vi "Autonomous Independent.vi"   [LabVIEW 2020]
doc: "This VI is called when autonomous begins, and will automatically be terminated when autonomous ends. You can carry out timed or sensor driven robot movement independently without needing to return to the caller."
uses:
  <vilib>/Rock Robotics/WPI/SafetyOutput/WPI_SafetyOutputConfigMenu.ctl
  <vilib>/Rock Robotics/WPI/Solenoid/WPI_SolenoidValue.ctl
  <vilib>/Rock Robotics/WPI/ThirdParty/REV Robotics/REVLib/Typedef/Spark MAX Control Type.ctl
  <vilib>/Rock Robotics/WPI/Utilities/WPI_GetSetVariantRefNum.vi
  <vilib>/Rock Robotics/Network Tables/NT Read String.vi
  <vilib>/Rock Robotics/Network Tables/NT Write Numeric Array.vi
  <vilib>/Rock Robotics/Network Tables/NT Read Number.vi
  Auto Variables.vi
  <vilib>/Rock Robotics/WPI/Solenoid/WPI_SolenoidSetEnum.vi
  Global Shooter Speed.vi
panel:
  # "Be sure to right-click and choose Data Operations>>Make Current Value default if you want to save the array values with the VI"
types:
  T1 = typedef "WPI_SafetyOutputConfigMenu.ctl" = enum16{"Enable", "Disable"}
  T2 = typedef "WPI_JoystickDevRef.ctl" = cluster{"Device":T3}
  T3 = typedef "WPI_JoystickDeviceEnum.ctl" = enum16{"USB 0", "USB 1", "USB 2", "USB 3", "USB 4", "USB 5"}
  T4 = typedef "WPI_RobotDriveDevRef.ctl" = cluster{"DevStatus":errorcluster, "Motors[]":T5[], "Square Inputs":bool, "Max Output":dbl}
  T5 = typedef "WPI_MotorControlDeviceRef.ctl" = cluster{"DeviceStatus":errorcluster, "Type":T6, "PWM":cluster{"PWM Channel":T7, "DeadBand":T8}, "CAN":cluster{"Device Number":u8, "SetOutput VI Ref":variant, "GetOutput VI Ref":variant, "Enable VI Ref":variant, "Disable VI Ref":variant, "Data":variant}, "Invert":bool, "DIO PWM":cluster{"PWM \"Enable\" Channel":T7, "DIOChannel":T9, "PWM Rate":dbl}}
  T6 = typedef "WPI_MotorControlType.ctl" = enum16{"PWM", "CAN", "DIO PWM"}
  T7 = typedef "FPGA_DIOPWMChannel.ctl" = enum8{"PWM 0", "PWM 1", "PWM 2", "PWM 3", "PWM 4", "PWM 5", "PWM 6", "PWM 7", "PWM 8", "PWM 9", "PWM MXP 0", "PWM MXP 1", "PWM MXP 2", "PWM MXP 3", "PWM MXP 4", "PWM MXP 5", "PWM MXP 6", "PWM MXP 7", "PWM MXP 8", "PWM MXP 9", "Invalid"}
  T8 = typedef "WPI_PWMDeadband.ctl" = cluster{"Name":string, "maxPositivePwm":i32, "minPositivePwm":i32, "centerPwm":i32, "maxNegativePwm":i32, "minNegativePwm":i32, "angularRange":u16}
  T9 = typedef "FPGA_DIOChannel.ctl" = enum8{"DIO 0", "DIO 1", "DIO 2", "DIO 3", "DIO 4", "DIO 5", "DIO 6", "DIO 7", "DIO 8", "DIO 9", "DIO MXP 0", "DIO MXP 1", "DIO MXP 2", "DIO MXP 3", "DIO MXP 4", "DIO MXP 5", "DIO MXP 6", "DIO MXP 7", "DIO MXP 8", "DIO MXP 9", "DIO MXP 10", "DIO MXP 11", "DIO MXP 12", "DIO MXP 13", "DIO MXP 14", "DIO MXP 15", "SPI Port CS1", "SPI Port CS2", "SPI Port CS3", "SPI Port MISO", "SPI Port MOSI", "Invalid"}
  T10 = typedef "WPI_SolenoidValue.ctl" = enum16{"Off", "On", "Forward", "Reverse"}
  T11 = typedef "Spark MAX Control Type.ctl" = enum16{"Percent VBus", "Voltage", "Velocity", "Position", "Smart Motion", "Current", "Smart Velocity"}
  T12 = typedef "WPI_SolenoidDevRef.ctl" = cluster{"DevStatus":errorcluster, "Pneumatics Control Module":u8, "Forward Solenoid Channel":T13, "Reverse Solenoid Channel":T13}
  T13 = typedef "WPI_SolenoidChannel.ctl" = enum8{"Solenoid 0", "Solenoid 1", "Solenoid 2", "Solenoid 3", "Solenoid 4", "Solenoid 5", "Solenoid 6", "Solenoid 7", "Solenoid 8", "Solenoid 9", "Solenoid 10", "Solenoid 11", "Solenoid 12", "Solenoid 13", "Solenoid 14", "Solenoid 15", "Invalid"}
  T14 = typedef "WPI_GyroDevRef.ctl" = cluster{"DevStatus":errorcluster, "Analog Channel":T15, "Gain (VoltsPerDegree/Second)":dbl, "Gyro Type":enum16{"Analog", "XRS450"}, "Handle":i32, "SPI Bus":T16, "Device Found":bool, "Sample Rate":dbl, "Calibrate On Open":bool, "Offset":dbl}
  T15 = typedef "FPGA_AIChannel.ctl" = enum8{"AI 0", "AI 1", "AI 2", "AI 3", "AI MXP 0", "AI MXP 1", "AI MXP 2", "AI MXP 3", "Invalid"}
  T16 = typedef "spi_bus.ctl" = enum16{"SPI On-Board, CS0", "SPI On-Board, CS1", "SPI On-Board, CS2", "SPI On-Board, CS3", "SPI MXP", "Invalid"}
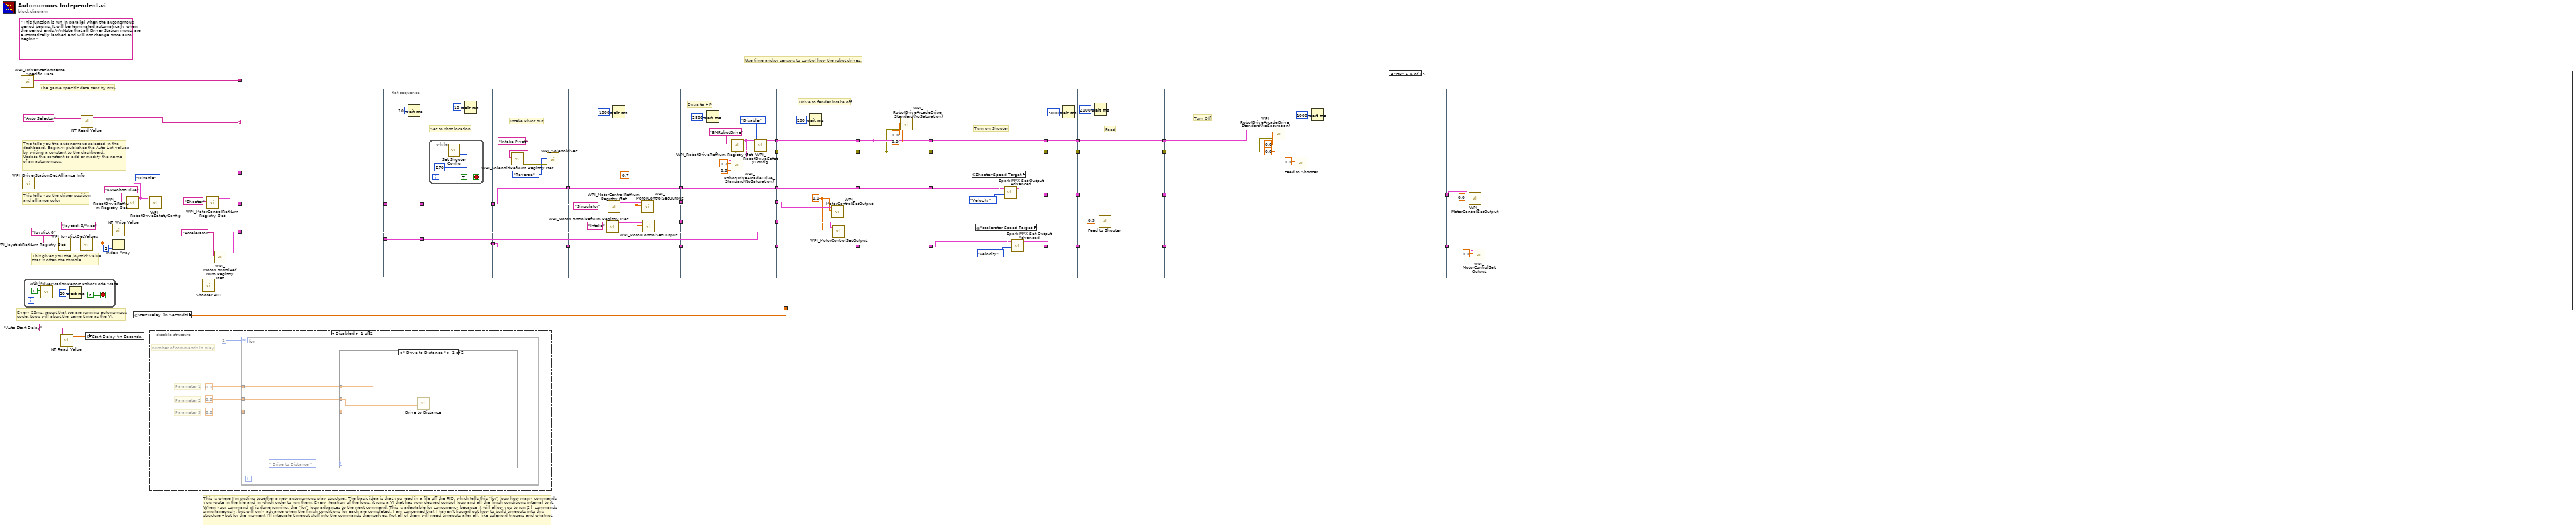
[diagram p0: block diagram]
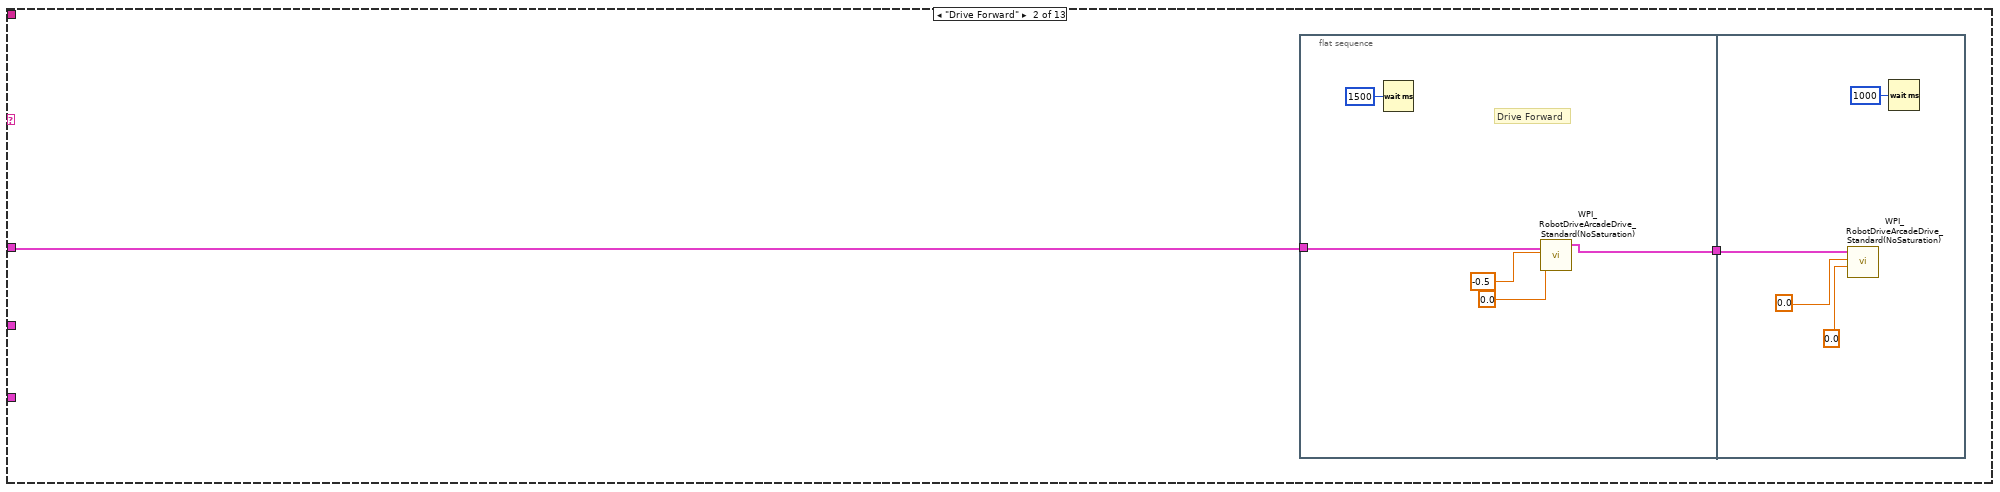
[diagram p5: hidden frame]
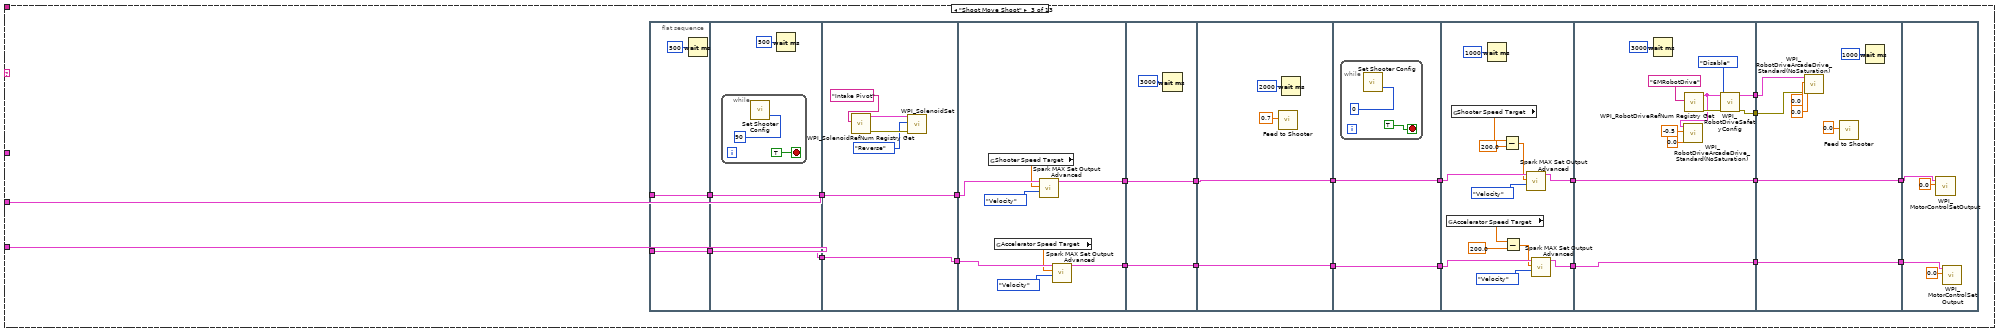
[diagram p6: hidden frame]
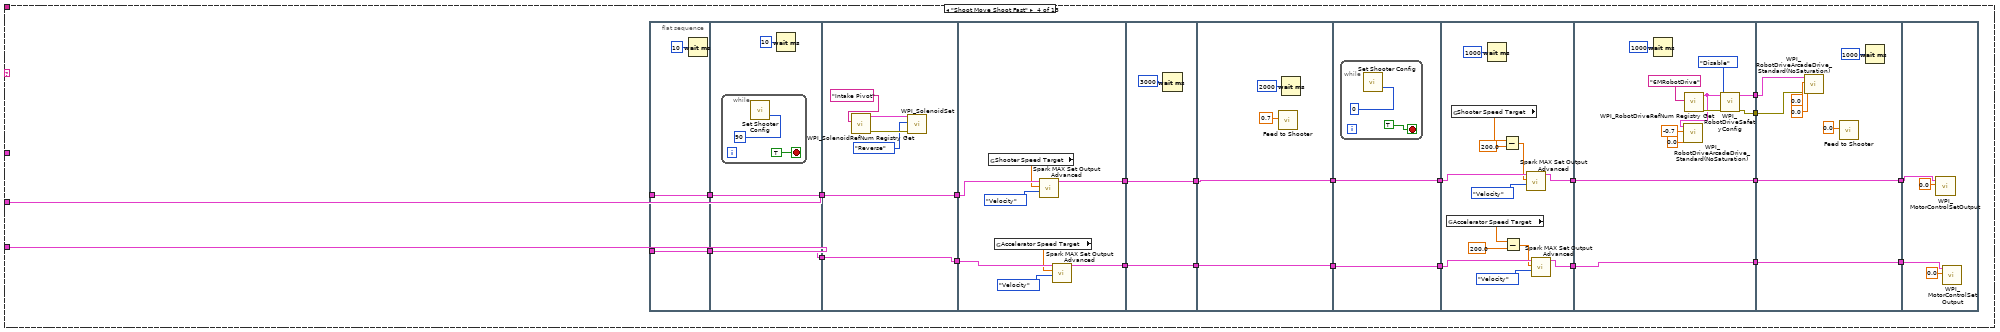
[diagram p7: hidden frame]
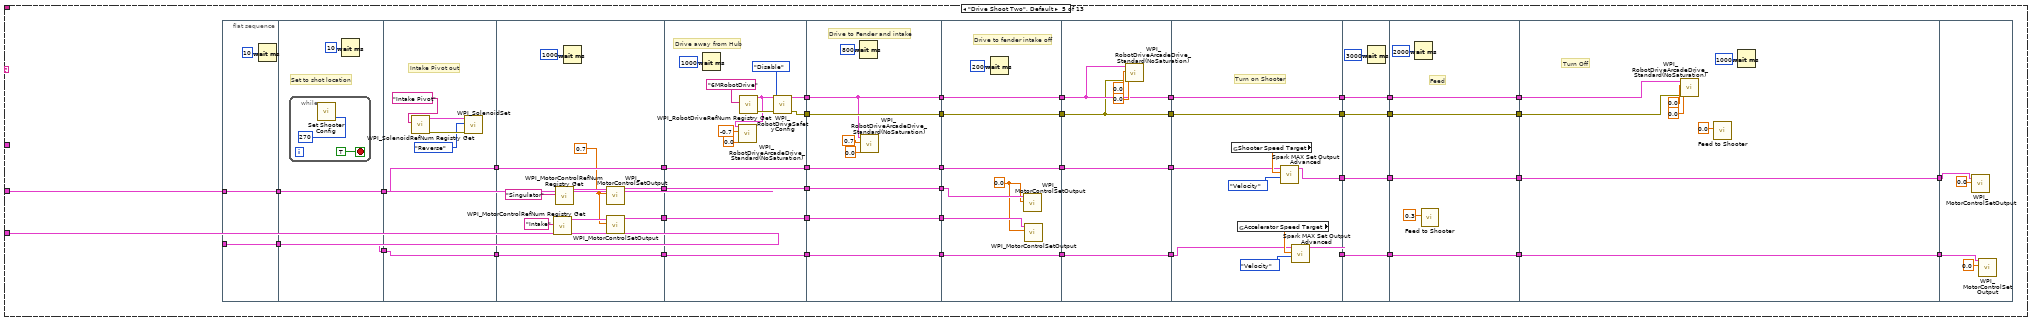
[diagram p8: hidden frame]
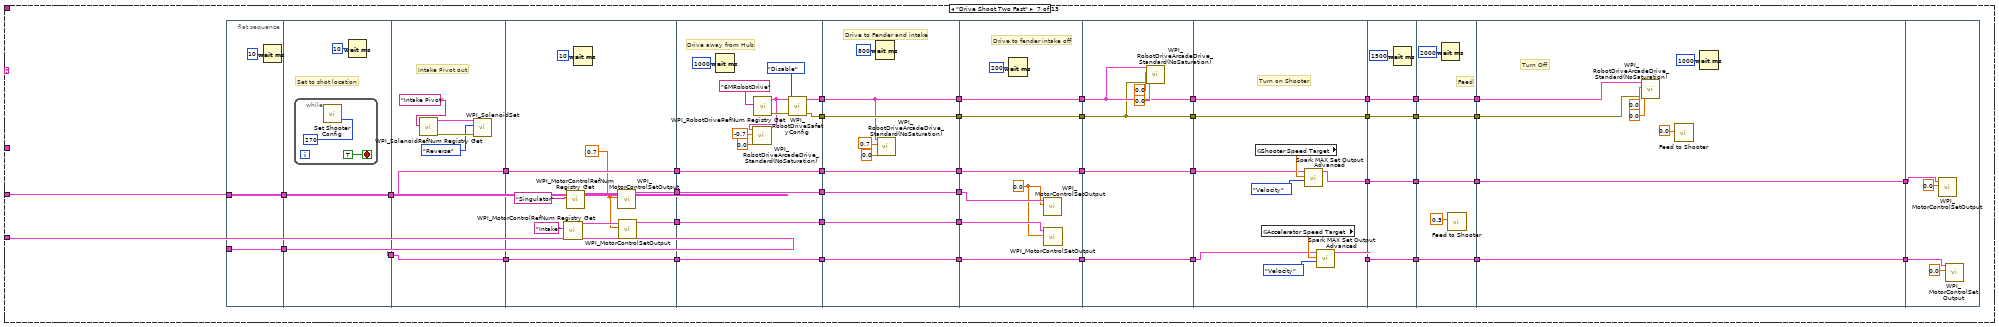
[diagram p9: hidden frame]
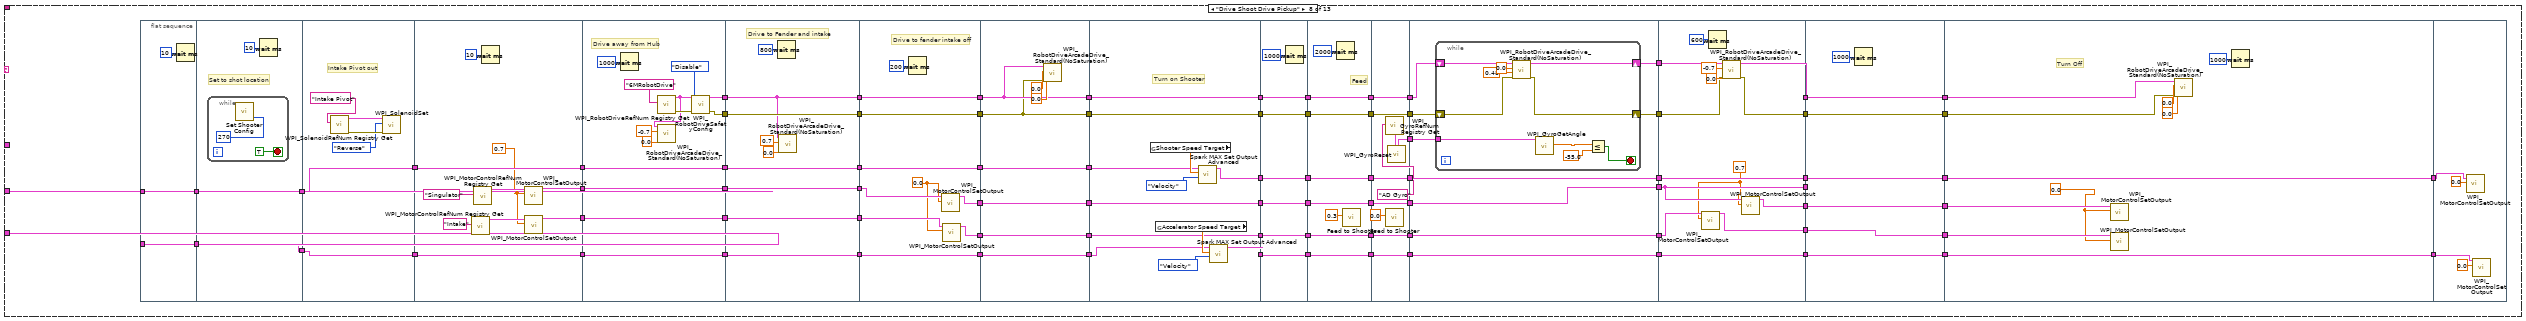
[diagram p10: hidden frame]
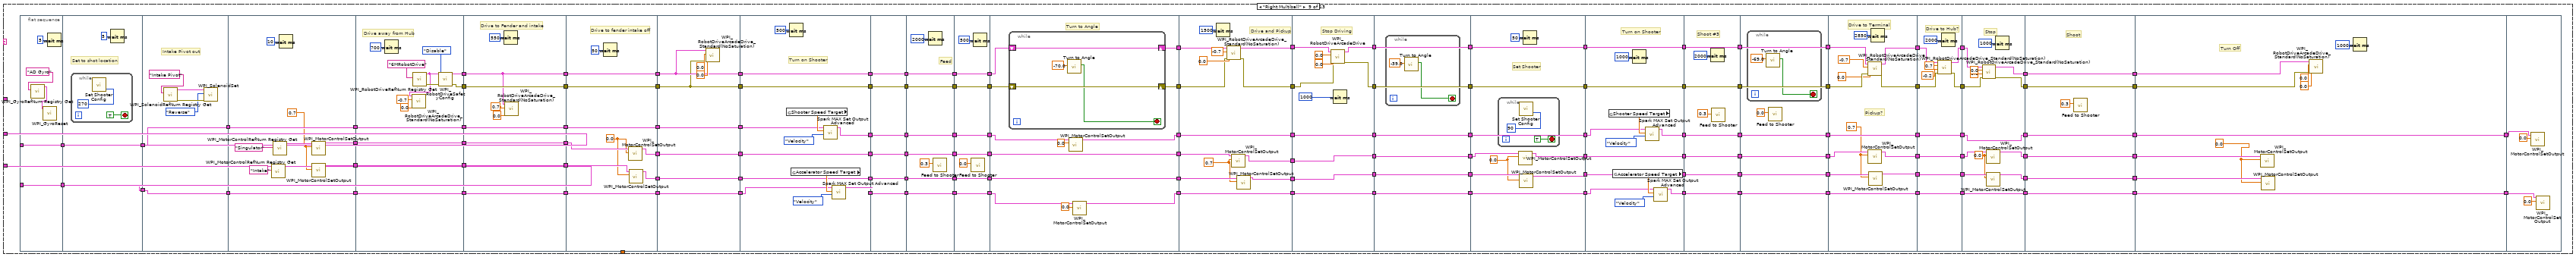
[diagram p11: hidden frame]
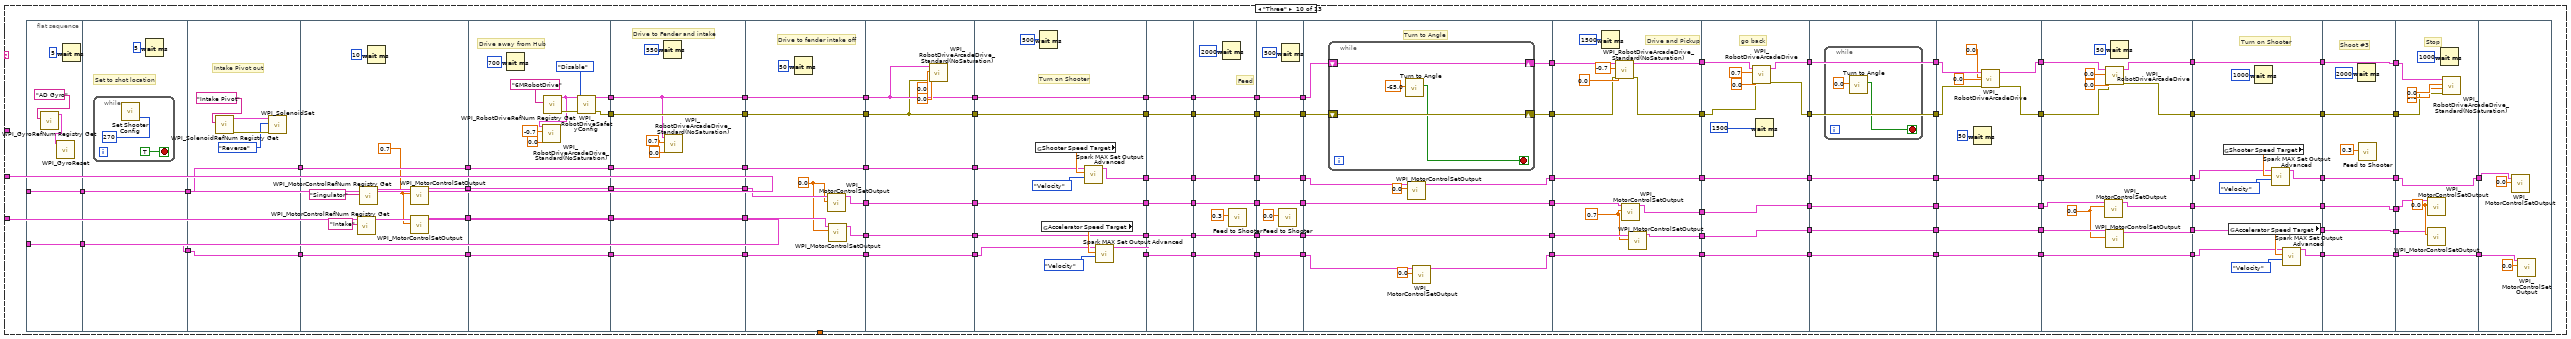
[diagram p12: hidden frame]
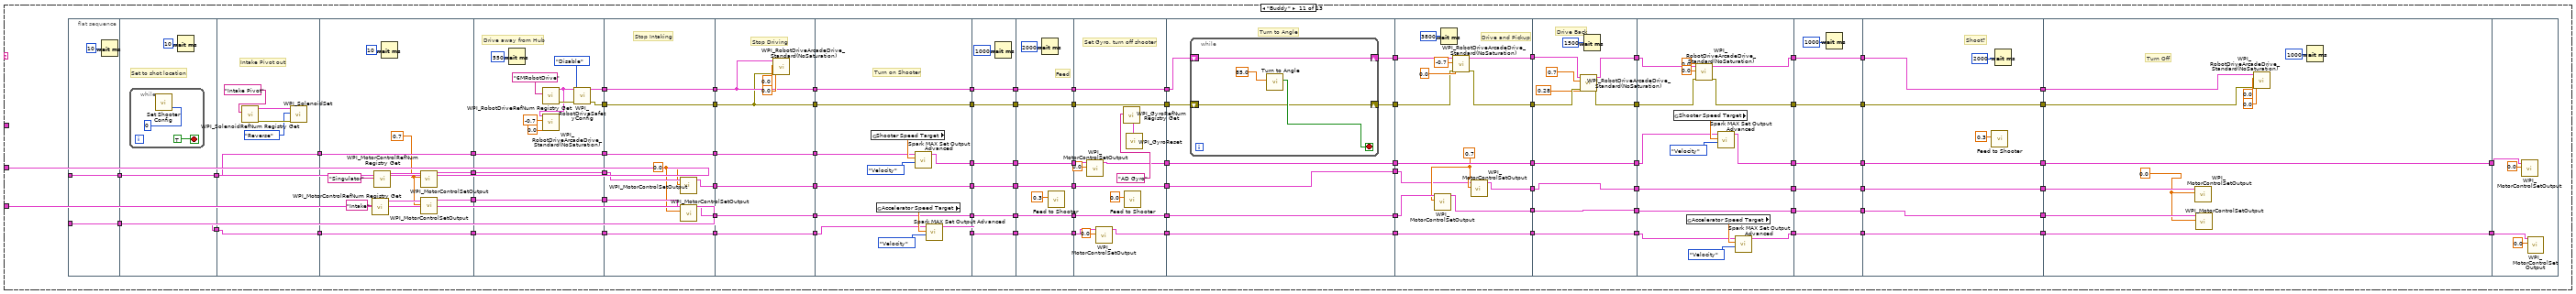
[diagram p13: hidden frame]
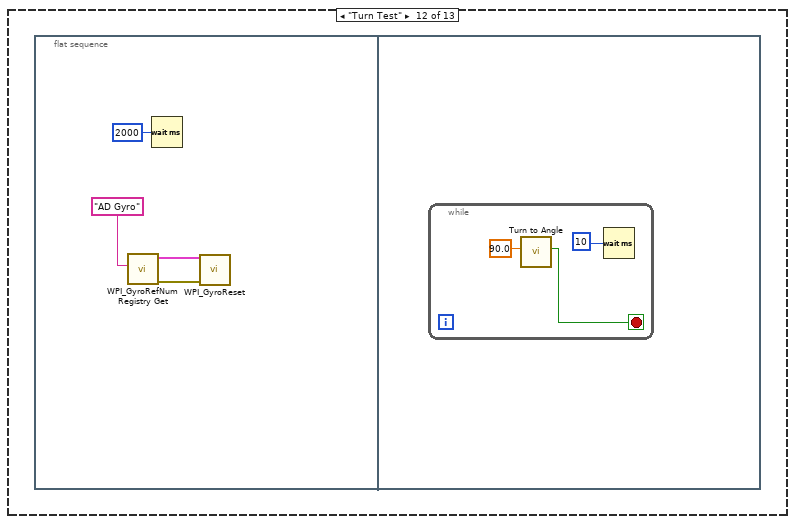
[diagram p14: hidden frame]
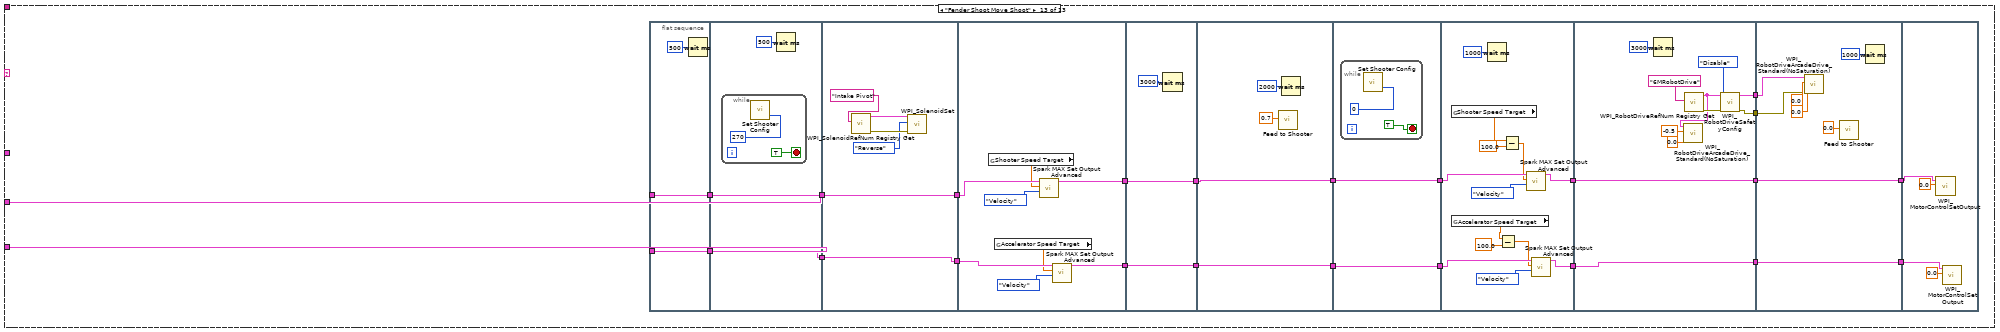
[diagram p15: hidden frame]
diagram:
  (unwired) "This function is run in parallel when the autonomous period begins. It will be terminated automatically when the period ends.\n\nNote that all Driver Station inputs are automatically latched and will not change once auto begins."
  # "This is where I'm putting together a new autonomous play structure. The basic idea is that you read in a file off the RIO, which tells this \"for\" loop how many commands\nyou wrote in the file and in which order to run them. Every iteration of the loop, it runs a VI that has your desired control loop and all the finish conditions internal to it.\nWhen your command VI is done running, the \"for\" loop advances to the next command. This is adaptable for concurrency because it will allow you to run 2+ commands\nsimultaneously, but will only advance when the finish conditions for each are completed. I am concerned that I haven't figured out how to build timeouts into this\nstructure - but for the moment I'll integrate timeout stuff into the commands themselves. Not all of them will need timeouts after all, like solenoid triggers and whatnot."
  # "The game specific data sent by FMS"
  # "This tells you the autonomous selected in the \ndashboard. Begin.vi publishes the Auto List values\nby writing a constant to the dashboard.\nUpdate the constant to add or modify the name\nof an autonomous."
  # "Every 20ms, report that we are running autonomous\ncode. Loop will abort the same time as the VI."
  # "This gives you the joystick value\nthat is often the throttle"
  # "Use time and/or sensors to control how the robot drives."
  # "This tells you the driver position\nand alliance color"
  n1 = call <vilib>:"WPI_DriverStationGame Specific Data.vi"() -> ("Game Specific Data"=w13:string)  [unwired: 11 in]
  n2 = call <vilib>:"WPI_DriverStationGet Alliance Info.vi"() -> ()  [unwired: 12 out]
  n3 = while {
    stop <- FALSE stop-if-true
    n4 = call <vilib>:"WPI_DriverStationReport Robot Code State.vi"("Autonomous"=TRUE) -> ()  [unwired: 10 in, 1 out]
    n5 = Wait (ms)(milliseconds to wait=u32 20) -> ()  [unwired: 1 out]
  }
  n6 = call <vilib>:"WPI_JoystickRefNum Registry Get.vi"("refnum name"="Joystick 0") -> ("JoystickDevRef"=w18:T2)  [unwired: 1 in, 9 out]
  n7 = call-poly <vilib>:"NT Read Value.vi"("Name"="Auto Start Delay") -> ("Numeric"=w10:dbl)  [unwired: 9 in, 1 out]
  n8 = call <vilib>:"WPI_JoystickGetValues.vi"("JoystickDevRef"=w18) -> ("Axes"=w15:dbl[])  [unwired: 6 in, 4 out]
  n9 = call-poly <vilib>:"NT Read Value.vi"("Name"="Auto Selector") -> ("String"=w1:string)  [unwired: 9 in, 1 out]
  n10 = global write "Auto Variables.vi" "Start Delay (in Seconds)"(w10) -> ()
  n11 = call-poly <vilib>:"NT Write Value.vi"("Numeric Array"=w15, "Name"="Joystick 0/Axes") -> ()  [unwired: 9 in, 1 out]
  n12 = Index Array(array=w15, index=2) -> ()  [unwired: 1 out]
  n13 = call <vilib>:"WPI_RobotDriveRefNum Registry Get.vi"("refnum name"="6MRobotDrive") -> ("error out"=w9:errorcluster, "RobotDriveDevRef"=w6:T4)  [unwired: 1 in, 8 out]
  n14 = global read "Auto Variables.vi" "Start Delay (in Seconds)"() -> (w12:dbl)
  n15 = disable-structure shown="Disabled" {
    frame Disabled {
      # "Parameter 3"
      # "Parameter 2"
      # "Parameter 1"
      # "number of commands in play"
      n16 = for {
        N: 1 -> [_]
        tunnel: 0.0 -> [w30]
        tunnel: 0.0 -> [w29]
        tunnel: 0.0 -> [w28]
        n17 = case shown="\" Drive to Distance \"" enum16{"No-op", " Drive to Distance "}." Drive to Distance " {
          tunnel: w30 -> [_ w32]
          tunnel: w29 -> [_ w31]
          tunnel: w28 -> [_ _]
          frame "No-op", Default {
          }
          frame " Drive to Distance " {
            n18 = call "Drive to Distance.vi"("Acceptable Error (in)"=w31, "Target in Inches"=w32) -> ()  [unwired: 9 in, 1 out]
          }
        }
      }
    }
    frame Enabled {
    }
  }
  n19 = call <vilib>:"WPI_RobotDriveSafetyConfig.vi"("error in (no error)"=w9, "mode"=WPI_SafetyOutputConfigMenu."Disable", "RobotDriveDevRef"=w6) -> ()  [unwired: 7 in, 2 out]
  n20 = call "Shooter PID.vi"() -> ()  [unwired: 12 in]
  n21 = call <vilib>:"WPI_MotorControlRefNum Registry Get.vi"("refnum name"="Shooter") -> ("MotorControlDevRef"=w5:T5)  [unwired: 9 in, 1 out]
  n22 = call <vilib>:"WPI_MotorControlRefNum Registry Get.vi"("refnum name"="Accelerator") -> ("MotorControlDevRef"=w4:T5)  [unwired: 9 in, 1 out]
  n23 = case shown="\"HP\"" w1 {
    tunnel: w13 -> [_ _ _ _ _ _ _ _ _ _ _ _ _]
    tunnel: w12 -> [_ _ _ _ _ _ _ _ _ _ _ _ _]
    tunnel: w6 -> [_ w34 _ _ _ _ _ _ _ _ _ _ _]
    tunnel: w5 -> [_ _ w64 w157 w274 w407 w537 w712 w1001 w1363 w1665 _ w1870]
    tunnel: w4 -> [_ _ w60 w153 w272 w405 w535 w710 w999 w1361 w1663 _ w1866]
    frame "Do Nothing" {
    }
    frame "Drive Forward" {
      n24 = flat-sequence {
        tunnel: w34 -> [w36]
        tunnel: [w35] -> w33
        tunnel: w33 -> [w40]
        frame #0 {
          # "Drive Forward"
          n25 = Wait (ms)(milliseconds to wait=u32 1500) -> ()  [unwired: 1 out]
          n26 = call <vilib>:"WPI_RobotDriveArcadeDrive_Standard(NoSaturation).vi"("Y axis value"=0.0, "X axis value"=-0.5, "RobotDriveDevRef"=w36) -> ("RobotDriveDevRef"=w35:T4)  [unwired: 1 in, 7 out]
        }
        frame #1 {
          n27 = call <vilib>:"WPI_RobotDriveArcadeDrive_Standard(NoSaturation).vi"("Y axis value"=0.0, "X axis value"=0.0, "RobotDriveDevRef"=w40) -> ()  [unwired: 1 in, 8 out]
          n28 = Wait (ms)(milliseconds to wait=u32 1000) -> ()  [unwired: 1 out]
        }
      }
    }
    frame "Shoot Move Shoot" {
      n29 = flat-sequence {
        tunnel: w60 -> [w69]
        tunnel: w64 -> [w70]
        tunnel: [w70] -> w45
        tunnel: [w69] -> w44
        tunnel: [w72] -> w65
        tunnel: [w71] -> w61
        tunnel: w45 -> [w72]
        tunnel: w44 -> [w71]
        tunnel: w65 -> [w77]
        tunnel: [w77] -> w63
        tunnel: [w76] -> w62
        tunnel: w61 -> [w76]
        tunnel: w63 -> [w89]
        tunnel: w62 -> [w88]
        tunnel: [w83] -> w49
        tunnel: [w82] -> w47
        tunnel: w49 -> [w92]
        tunnel: [w92] -> w48
        tunnel: w47 -> [w91]
        tunnel: [w91] -> w46
        tunnel: [w95] -> w53
        tunnel: w48 -> [w95]
        tunnel: [w94] -> w51
        tunnel: w46 -> [w94]
        tunnel: w53 -> [w98]
        tunnel: [w98] -> w52
        tunnel: w51 -> [w97]
        tunnel: [w97] -> w50
        tunnel: w52 -> [w111]
        tunnel: [w110] -> w57
        tunnel: w50 -> [w108]
        tunnel: [w107] -> w56
        tunnel: [w118] -> w67
        tunnel: [w117] -> w66
        tunnel: w57 -> [w115]
        tunnel: w56 -> [w114]
        tunnel: [w115] -> w59
        tunnel: [w114] -> w58
        tunnel: w67 -> [w129]
        tunnel: w66 -> [w128]
        tunnel: w59 -> [w125]
        tunnel: w58 -> [w126]
        tunnel: [w126] -> w55
        tunnel: [w125] -> w54
        tunnel: w55 -> [w135]
        tunnel: w54 -> [w133]
        frame #0 {
          n30 = Wait (ms)(milliseconds to wait=u32 500) -> ()  [unwired: 1 out]
        }
        frame #1 {
          n31 = while {
            stop <- TRUE stop-if-true
            n32 = call "Set Shooter Config.vi"("POV Joystick Input"=90) -> ()  [unwired: 3 in]
          }
          n33 = Wait (ms)(milliseconds to wait=u32 500) -> ()  [unwired: 1 out]
        }
        frame #2 {
          n34 = call <vilib>:"WPI_SolenoidRefNum Registry Get.vi"("refnum name"="Intake Pivot") -> ("error out"=w81:errorcluster, "SolenoidDevRef"=w80:T12)  [unwired: 9 in]
          n35 = call-poly <vilib>:"WPI_SolenoidSet.vi"("error in (no error)"=w81, "Value"=WPI_SolenoidValue."Reverse", "SolenoidDevRef"=w80) -> ()  [unwired: 7 in, 2 out]
        }
        frame #3 {
          n36 = global read "Global Shooter Speed.vi" "Shooter Speed Target"() -> (w86:dbl)
          n37 = global read "Global Shooter Speed.vi" "Accelerator Speed Target"() -> (w84:dbl)
          n38 = call <vilib>:"Spark MAX Set Output Advanced.vi"("Control Mode"=Spark_MAX_Control_Type."Velocity", "Setpoint"=w86, "MotorControlDevRef"=w89) -> ("MotorControlDevRef"=w83:T5)  [unwired: 7 in, 1 out]
          n39 = call <vilib>:"Spark MAX Set Output Advanced.vi"("Control Mode"=Spark_MAX_Control_Type."Velocity", "Setpoint"=w84, "MotorControlDevRef"=w88) -> ("MotorControlDevRef"=w82:T5)  [unwired: 7 in, 1 out]
        }
        frame #4 {
          n40 = Wait (ms)(milliseconds to wait=u32 3000) -> ()  [unwired: 1 out]
        }
        frame #5 {
          n41 = call "Feed to Shooter.vi"("Feed Input"=0.7) -> ()  [unwired: 11 in]
          n42 = Wait (ms)(milliseconds to wait=u32 2000) -> ()  [unwired: 1 out]
        }
        frame #6 {
          n43 = while {
            stop <- TRUE stop-if-true
            n44 = call "Set Shooter Config.vi"("POV Joystick Input"=0) -> ()  [unwired: 3 in]
          }
        }
        frame #7 {
          n45 = global read "Global Shooter Speed.vi" "Accelerator Speed Target"() -> (w102:dbl)
          n46 = global read "Global Shooter Speed.vi" "Shooter Speed Target"() -> (w106:dbl)
          n47 = Wait (ms)(milliseconds to wait=u32 1000) -> ()  [unwired: 1 out]
          n48 = Subtract(x=w106, y=200.0) -> (x-y=w104:dbl)
          n49 = Subtract(x=w102, y=200.0) -> (x-y=w103:dbl)
          n50 = call <vilib>:"Spark MAX Set Output Advanced.vi"("Control Mode"=Spark_MAX_Control_Type."Velocity", "Setpoint"=w104, "MotorControlDevRef"=w111) -> ("MotorControlDevRef"=w110:T5)  [unwired: 7 in, 1 out]
          n51 = call <vilib>:"Spark MAX Set Output Advanced.vi"("Control Mode"=Spark_MAX_Control_Type."Velocity", "Setpoint"=w103, "MotorControlDevRef"=w108) -> ("MotorControlDevRef"=w107:T5)  [unwired: 7 in, 1 out]
        }
        frame #8 {
          n52 = Wait (ms)(milliseconds to wait=u32 3000) -> ()  [unwired: 1 out]
          n53 = call <vilib>:"WPI_RobotDriveRefNum Registry Get.vi"("refnum name"="6MRobotDrive") -> ("error out"=w121:errorcluster, "RobotDriveDevRef"=w120:T4)  [unwired: 1 in, 8 out]
          n54 = call <vilib>:"WPI_RobotDriveArcadeDrive_Standard(NoSaturation).vi"("Y axis value"=0.0, "X axis value"=-0.5, "RobotDriveDevRef"=w120) -> ()  [unwired: 1 in, 8 out]
          n55 = call <vilib>:"WPI_RobotDriveSafetyConfig.vi"("error in (no error)"=w121, "mode"=WPI_SafetyOutputConfigMenu."Disable", "RobotDriveDevRef"=w120) -> ("error out"=w117:errorcluster, "RobotDriveDevRef"=w118:T4)  [unwired: 7 in]
        }
        frame #9 {
          n56 = call <vilib>:"WPI_RobotDriveArcadeDrive_Standard(NoSaturation).vi"("error in (no error)"=w128, "Y axis value"=0.0, "X axis value"=0.0, "RobotDriveDevRef"=w129) -> ()  [unwired: 8 out]
          n57 = call "Feed to Shooter.vi"("Feed Input"=0.0) -> ()  [unwired: 11 in]
          n58 = Wait (ms)(milliseconds to wait=u32 1000) -> ()  [unwired: 1 out]
        }
        frame #10 {
          n59 = call <vilib>:"WPI_MotorControlSetOutput.vi"("Output"=0.0, "MotorControlDevRef"=w133) -> ()  [unwired: 7 in, 3 out]
          n60 = call <vilib>:"WPI_MotorControlSetOutput.vi"("Output"=0.0, "MotorControlDevRef"=w135) -> ()  [unwired: 7 in, 3 out]
        }
      }
    }
    frame "Shoot Move Shoot Fast" {
      n61 = flat-sequence {
        tunnel: w153 -> [w162]
        tunnel: w157 -> [w163]
        tunnel: [w163] -> w138
        tunnel: [w162] -> w137
        tunnel: [w165] -> w158
        tunnel: [w164] -> w154
        tunnel: w138 -> [w165]
        tunnel: w137 -> [w164]
        tunnel: w158 -> [w170]
        tunnel: [w170] -> w156
        tunnel: [w169] -> w155
        tunnel: w154 -> [w169]
        tunnel: w156 -> [w182]
        tunnel: w155 -> [w181]
        tunnel: [w176] -> w142
        tunnel: [w175] -> w140
        tunnel: w142 -> [w185]
        tunnel: [w185] -> w141
        tunnel: w140 -> [w184]
        tunnel: [w184] -> w139
        tunnel: [w188] -> w146
        tunnel: w141 -> [w188]
        tunnel: [w187] -> w144
        tunnel: w139 -> [w187]
        tunnel: w146 -> [w191]
        tunnel: [w191] -> w145
        tunnel: w144 -> [w190]
        tunnel: [w190] -> w143
        tunnel: w145 -> [w204]
        tunnel: [w203] -> w150
        tunnel: w143 -> [w201]
        tunnel: [w200] -> w149
        tunnel: [w211] -> w160
        tunnel: [w210] -> w159
        tunnel: w150 -> [w208]
        tunnel: w149 -> [w207]
        tunnel: [w208] -> w152
        tunnel: [w207] -> w151
        tunnel: w160 -> [w222]
        tunnel: w159 -> [w221]
        tunnel: w152 -> [w218]
        tunnel: w151 -> [w219]
        tunnel: [w219] -> w148
        tunnel: [w218] -> w147
        tunnel: w148 -> [w228]
        tunnel: w147 -> [w226]
        frame #0 {
          n62 = Wait (ms)(milliseconds to wait=u32 10) -> ()  [unwired: 1 out]
        }
        frame #1 {
          n63 = while {
            stop <- TRUE stop-if-true
            n64 = call "Set Shooter Config.vi"("POV Joystick Input"=90) -> ()  [unwired: 3 in]
          }
          n65 = Wait (ms)(milliseconds to wait=u32 10) -> ()  [unwired: 1 out]
        }
        frame #2 {
          n66 = call <vilib>:"WPI_SolenoidRefNum Registry Get.vi"("refnum name"="Intake Pivot") -> ("error out"=w174:errorcluster, "SolenoidDevRef"=w173:T12)  [unwired: 9 in]
          n67 = call-poly <vilib>:"WPI_SolenoidSet.vi"("error in (no error)"=w174, "Value"=WPI_SolenoidValue."Reverse", "SolenoidDevRef"=w173) -> ()  [unwired: 7 in, 2 out]
        }
        frame #3 {
          n68 = global read "Global Shooter Speed.vi" "Shooter Speed Target"() -> (w179:dbl)
          n69 = global read "Global Shooter Speed.vi" "Accelerator Speed Target"() -> (w177:dbl)
          n70 = call <vilib>:"Spark MAX Set Output Advanced.vi"("Control Mode"=Spark_MAX_Control_Type."Velocity", "Setpoint"=w179, "MotorControlDevRef"=w182) -> ("MotorControlDevRef"=w176:T5)  [unwired: 7 in, 1 out]
          n71 = call <vilib>:"Spark MAX Set Output Advanced.vi"("Control Mode"=Spark_MAX_Control_Type."Velocity", "Setpoint"=w177, "MotorControlDevRef"=w181) -> ("MotorControlDevRef"=w175:T5)  [unwired: 7 in, 1 out]
        }
        frame #4 {
          n72 = Wait (ms)(milliseconds to wait=u32 3000) -> ()  [unwired: 1 out]
        }
        frame #5 {
          n73 = call "Feed to Shooter.vi"("Feed Input"=0.7) -> ()  [unwired: 11 in]
          n74 = Wait (ms)(milliseconds to wait=u32 2000) -> ()  [unwired: 1 out]
        }
        frame #6 {
          n75 = while {
            stop <- TRUE stop-if-true
            n76 = call "Set Shooter Config.vi"("POV Joystick Input"=0) -> ()  [unwired: 3 in]
          }
        }
        frame #7 {
          n77 = global read "Global Shooter Speed.vi" "Accelerator Speed Target"() -> (w195:dbl)
          n78 = global read "Global Shooter Speed.vi" "Shooter Speed Target"() -> (w199:dbl)
          n79 = Wait (ms)(milliseconds to wait=u32 1000) -> ()  [unwired: 1 out]
          n80 = Subtract(x=w199, y=200.0) -> (x-y=w197:dbl)
          n81 = Subtract(x=w195, y=200.0) -> (x-y=w196:dbl)
          n82 = call <vilib>:"Spark MAX Set Output Advanced.vi"("Control Mode"=Spark_MAX_Control_Type."Velocity", "Setpoint"=w197, "MotorControlDevRef"=w204) -> ("MotorControlDevRef"=w203:T5)  [unwired: 7 in, 1 out]
          n83 = call <vilib>:"Spark MAX Set Output Advanced.vi"("Control Mode"=Spark_MAX_Control_Type."Velocity", "Setpoint"=w196, "MotorControlDevRef"=w201) -> ("MotorControlDevRef"=w200:T5)  [unwired: 7 in, 1 out]
        }
        frame #8 {
          n84 = Wait (ms)(milliseconds to wait=u32 1000) -> ()  [unwired: 1 out]
          n85 = call <vilib>:"WPI_RobotDriveRefNum Registry Get.vi"("refnum name"="6MRobotDrive") -> ("error out"=w214:errorcluster, "RobotDriveDevRef"=w213:T4)  [unwired: 1 in, 8 out]
          n86 = call <vilib>:"WPI_RobotDriveArcadeDrive_Standard(NoSaturation).vi"("Y axis value"=0.0, "X axis value"=-0.7, "RobotDriveDevRef"=w213) -> ()  [unwired: 1 in, 8 out]
          n87 = call <vilib>:"WPI_RobotDriveSafetyConfig.vi"("error in (no error)"=w214, "mode"=WPI_SafetyOutputConfigMenu."Disable", "RobotDriveDevRef"=w213) -> ("error out"=w210:errorcluster, "RobotDriveDevRef"=w211:T4)  [unwired: 7 in]
        }
        frame #9 {
          n88 = call <vilib>:"WPI_RobotDriveArcadeDrive_Standard(NoSaturation).vi"("error in (no error)"=w221, "Y axis value"=0.0, "X axis value"=0.0, "RobotDriveDevRef"=w222) -> ()  [unwired: 8 out]
          n89 = call "Feed to Shooter.vi"("Feed Input"=0.0) -> ()  [unwired: 11 in]
          n90 = Wait (ms)(milliseconds to wait=u32 1000) -> ()  [unwired: 1 out]
        }
        frame #10 {
          n91 = call <vilib>:"WPI_MotorControlSetOutput.vi"("Output"=0.0, "MotorControlDevRef"=w226) -> ()  [unwired: 7 in, 3 out]
          n92 = call <vilib>:"WPI_MotorControlSetOutput.vi"("Output"=0.0, "MotorControlDevRef"=w228) -> ()  [unwired: 7 in, 3 out]
        }
      }
    }
    frame "Drive Shoot Two", Default {
      n93 = flat-sequence {
        tunnel: w272 -> [w277]
        tunnel: w274 -> [w278]
        tunnel: [w278] -> w269
        tunnel: [w277] -> w268
        tunnel: [w280] -> w275
        tunnel: [w279] -> w273
        tunnel: w269 -> [w280]
        tunnel: w268 -> [w279]
        tunnel: w275 -> [w285]
        tunnel: w273 -> [w284]
        tunnel: [w285] -> w263
        tunnel: [w284] -> w260
        tunnel: [w299] -> w264
        tunnel: w263 -> [w299]
        tunnel: [w298] -> w261
        tunnel: w260 -> [w298]
        tunnel: [w293] -> w254
        tunnel: [w292] -> w252
        tunnel: [w306] -> w267
        tunnel: [w305] -> w266
        tunnel: [w303] -> w265
        tunnel: w264 -> [w303]
        tunnel: [w302] -> w262
        tunnel: w261 -> [w302]
        tunnel: [w301] -> w255
        tunnel: w254 -> [w301]
        tunnel: [w300] -> w253
        tunnel: w252 -> [w300]
        tunnel: w267 -> [w318]
        tunnel: [w318] -> w239
        tunnel: w266 -> [w321]
        tunnel: [w321] -> w237
        tunnel: [w315] -> w235
        tunnel: [w316] -> w233
        tunnel: w265 -> [w316]
        tunnel: w262 -> [w315]
        tunnel: w255 -> [w313]
        tunnel: w253 -> [w314]
        tunnel: [w314] -> w231
        tunnel: [w313] -> w230
        tunnel: w239 -> [w329]
        tunnel: [w329] -> w238
        tunnel: w237 -> [w328]
        tunnel: [w328] -> w236
        tunnel: w235 -> [w327]
        tunnel: [w327] -> w234
        tunnel: w233 -> [w326]
        tunnel: [w326] -> w232
        tunnel: w231 -> [w325]
        tunnel: w230 -> [w324]
        tunnel: w238 -> [w331]
        tunnel: [w331] -> w243
        tunnel: w236 -> [w330]
        tunnel: [w330] -> w242
        tunnel: w234 -> [w335]
        tunnel: [w335] -> w241
        tunnel: w232 -> [w334]
        tunnel: [w334] -> w240
        tunnel: w243 -> [w345]
        tunnel: [w345] -> w251
        tunnel: w242 -> [w344]
        tunnel: [w344] -> w249
        tunnel: [w336] -> w247
        tunnel: w241 -> [w339]
        tunnel: [w338] -> w245
        tunnel: w240 -> [w337]
        tunnel: w251 -> [w350]
        tunnel: [w350] -> w250
        tunnel: w249 -> [w349]
        tunnel: [w349] -> w248
        tunnel: w247 -> [w348]
        tunnel: [w348] -> w246
        tunnel: w245 -> [w347]
        tunnel: [w347] -> w244
        tunnel: w250 -> [w356]
        tunnel: [w356] -> w259
        tunnel: w248 -> [w355]
        tunnel: [w355] -> w258
        tunnel: w246 -> [w354]
        tunnel: [w354] -> w257
        tunnel: w244 -> [w353]
        tunnel: [w353] -> w256
        tunnel: w259 -> [w361]
        tunnel: w258 -> [w360]
        tunnel: w257 -> [w357]
        tunnel: w256 -> [w358]
        tunnel: [w358] -> w271
        tunnel: [w357] -> w270
        tunnel: w271 -> [w367]
        tunnel: w270 -> [w365]
        frame #0 {
          n94 = Wait (ms)(milliseconds to wait=u32 10) -> ()  [unwired: 1 out]
        }
        frame #1 {
          # "Set to shot location"
          n95 = while {
            stop <- TRUE stop-if-true
            n96 = call "Set Shooter Config.vi"("POV Joystick Input"=270) -> ()  [unwired: 3 in]
          }
          n97 = Wait (ms)(milliseconds to wait=u32 10) -> ()  [unwired: 1 out]
        }
        frame #2 {
          # "Intake Pivot out"
          n98 = call <vilib>:"WPI_SolenoidRefNum Registry Get.vi"("refnum name"="Intake Pivot") -> ("error out"=w289:errorcluster, "SolenoidDevRef"=w288:T12)  [unwired: 9 in]
          n99 = call-poly <vilib>:"WPI_SolenoidSet.vi"("error in (no error)"=w289, "Value"=WPI_SolenoidValue."Reverse", "SolenoidDevRef"=w288) -> ()  [unwired: 7 in, 2 out]
        }
        frame #3 {
          w291 = 0.7 ("Output")
          n100 = call <vilib>:"WPI_MotorControlRefNum Registry Get.vi"("refnum name"="Intake") -> ("MotorControlDevRef"=w294:T5)  [unwired: 9 in, 1 out]
          n101 = call <vilib>:"WPI_MotorControlRefNum Registry Get.vi"("refnum name"="Singulator") -> ("MotorControlDevRef"=w295:T5)  [unwired: 9 in, 1 out]
          n102 = Wait (ms)(milliseconds to wait=u32 1000) -> ()  [unwired: 1 out]
          n103 = call <vilib>:"WPI_MotorControlSetOutput.vi"("Output"=w291, "MotorControlDevRef"=w295) -> ("MotorControlDevRef"=w293:T5)  [unwired: 7 in, 2 out]
          n104 = call <vilib>:"WPI_MotorControlSetOutput.vi"("Output"=w291, "MotorControlDevRef"=w294) -> ("MotorControlDevRef"=w292:T5)  [unwired: 7 in, 2 out]
        }
        frame #4 {
          # "Drive away from Hub"
          n105 = Wait (ms)(milliseconds to wait=u32 1000) -> ()  [unwired: 1 out]
          n106 = call <vilib>:"WPI_RobotDriveRefNum Registry Get.vi"("refnum name"="6MRobotDrive") -> ("error out"=w309:errorcluster, "RobotDriveDevRef"=w308:T4)  [unwired: 1 in, 8 out]
          n107 = call <vilib>:"WPI_RobotDriveArcadeDrive_Standard(NoSaturation).vi"("Y axis value"=0.0, "X axis value"=-0.7, "RobotDriveDevRef"=w308) -> ()  [unwired: 1 in, 8 out]
          n108 = call <vilib>:"WPI_RobotDriveSafetyConfig.vi"("error in (no error)"=w309, "mode"=WPI_SafetyOutputConfigMenu."Disable", "RobotDriveDevRef"=w308) -> ("error out"=w305:errorcluster, "RobotDriveDevRef"=w306:T4)  [unwired: 7 in]
        }
        frame #5 {
          # "Drive to Fender and intake"
          n109 = Wait (ms)(milliseconds to wait=u32 800) -> ()  [unwired: 1 out]
          n110 = call <vilib>:"WPI_RobotDriveArcadeDrive_Standard(NoSaturation).vi"("Y axis value"=0.0, "X axis value"=0.7, "RobotDriveDevRef"=w318) -> ()  [unwired: 1 in, 8 out]
        }
        frame #6 {
          w323 = 0.0 ("Output")
          # "Drive to fender intake off"
          n111 = Wait (ms)(milliseconds to wait=u32 200) -> ()  [unwired: 1 out]
          n112 = call <vilib>:"WPI_MotorControlSetOutput.vi"("Output"=w323, "MotorControlDevRef"=w324) -> ()  [unwired: 7 in, 3 out]
          n113 = call <vilib>:"WPI_MotorControlSetOutput.vi"("Output"=w323, "MotorControlDevRef"=w325) -> ()  [unwired: 7 in, 3 out]
        }
        frame #7 {
          n114 = call <vilib>:"WPI_RobotDriveArcadeDrive_Standard(NoSaturation).vi"("error in (no error)"=w330, "Y axis value"=0.0, "X axis value"=0.0, "RobotDriveDevRef"=w331) -> ()  [unwired: 8 out]
        }
        frame #8 {
          # "Turn on Shooter"
          n115 = global read "Global Shooter Speed.vi" "Shooter Speed Target"() -> (w342:dbl)
          n116 = global read "Global Shooter Speed.vi" "Accelerator Speed Target"() -> (w340:dbl)
          n117 = call <vilib>:"Spark MAX Set Output Advanced.vi"("Control Mode"=Spark_MAX_Control_Type."Velocity", "Setpoint"=w342, "MotorControlDevRef"=w337) -> ("MotorControlDevRef"=w336:T5)  [unwired: 7 in, 1 out]
          n118 = call <vilib>:"Spark MAX Set Output Advanced.vi"("Control Mode"=Spark_MAX_Control_Type."Velocity", "Setpoint"=w340, "MotorControlDevRef"=w339) -> ("MotorControlDevRef"=w338:T5)  [unwired: 7 in, 1 out]
        }
        frame #9 {
          n119 = Wait (ms)(milliseconds to wait=u32 3000) -> ()  [unwired: 1 out]
        }
        frame #10 {
          # "Feed"
          n120 = Wait (ms)(milliseconds to wait=u32 2000) -> ()  [unwired: 1 out]
          n121 = call "Feed to Shooter.vi"("Feed Input"=0.3) -> ()  [unwired: 11 in]
        }
        frame #11 {
          # "Turn Off"
          n122 = call <vilib>:"WPI_RobotDriveArcadeDrive_Standard(NoSaturation).vi"("error in (no error)"=w360, "Y axis value"=0.0, "X axis value"=0.0, "RobotDriveDevRef"=w361) -> ()  [unwired: 8 out]
          n123 = call "Feed to Shooter.vi"("Feed Input"=0.0) -> ()  [unwired: 11 in]
          n124 = Wait (ms)(milliseconds to wait=u32 1000) -> ()  [unwired: 1 out]
        }
        frame #12 {
          n125 = call <vilib>:"WPI_MotorControlSetOutput.vi"("Output"=0.0, "MotorControlDevRef"=w365) -> ()  [unwired: 7 in, 3 out]
          n126 = call <vilib>:"WPI_MotorControlSetOutput.vi"("Output"=0.0, "MotorControlDevRef"=w367) -> ()  [unwired: 7 in, 3 out]
        }
      }
    }
    frame "HP" {
      n127 = flat-sequence {
        tunnel: w405 -> [w410]
        tunnel: w407 -> [w411]
        tunnel: [w411] -> w402
        tunnel: [w410] -> w401
        tunnel: [w413] -> w408
        tunnel: [w412] -> w406
        tunnel: w402 -> [w413]
        tunnel: w401 -> [w412]
        tunnel: w408 -> [w418]
        tunnel: w406 -> [w417]
        tunnel: [w418] -> w399
        tunnel: [w417] -> w397
        tunnel: [w432] -> w400
        tunnel: w399 -> [w432]
        tunnel: [w431] -> w398
        tunnel: w397 -> [w431]
        tunnel: [w426] -> w392
        tunnel: [w425] -> w391
        tunnel: [w439] -> w374
        tunnel: [w437] -> w372
        tunnel: w400 -> [w437]
        tunnel: [w436] -> w373
        tunnel: w398 -> [w436]
        tunnel: [w435] -> w371
        tunnel: w392 -> [w435]
        tunnel: [w434] -> w370
        tunnel: w391 -> [w434]
        tunnel: [w433] -> w369
        tunnel: [w446] -> w378
        tunnel: w374 -> [w453]
        tunnel: [w453] -> w377
        tunnel: w373 -> [w452]
        tunnel: [w452] -> w376
        tunnel: w372 -> [w451]
        tunnel: [w451] -> w375
        tunnel: w370 -> [w450]
        tunnel: w371 -> [w449]
        tunnel: w369 -> [w446]
        tunnel: w378 -> [w455]
        tunnel: [w455] -> w382
        tunnel: w377 -> [w454]
        tunnel: [w454] -> w381
        tunnel: w376 -> [w459]
        tunnel: [w459] -> w380
        tunnel: w375 -> [w458]
        tunnel: [w458] -> w379
        tunnel: w382 -> [w469]
        tunnel: [w469] -> w390
        tunnel: w381 -> [w468]
        tunnel: [w468] -> w388
        tunnel: [w460] -> w386
        tunnel: w380 -> [w463]
        tunnel: [w462] -> w384
        tunnel: w379 -> [w461]
        tunnel: w390 -> [w474]
        tunnel: [w474] -> w389
        tunnel: w388 -> [w473]
        tunnel: [w473] -> w387
        tunnel: w386 -> [w472]
        tunnel: [w472] -> w385
        tunnel: w384 -> [w471]
        tunnel: [w471] -> w383
        tunnel: w389 -> [w480]
        tunnel: [w480] -> w396
        tunnel: w387 -> [w479]
        tunnel: [w479] -> w395
        tunnel: w385 -> [w478]
        tunnel: [w478] -> w394
        tunnel: w383 -> [w477]
        tunnel: [w477] -> w393
        tunnel: w396 -> [w485]
        tunnel: w395 -> [w484]
        tunnel: w394 -> [w481]
        tunnel: w393 -> [w482]
        tunnel: [w482] -> w404
        tunnel: [w481] -> w403
        tunnel: w404 -> [w491]
        tunnel: w403 -> [w489]
        frame #0 {
          n128 = Wait (ms)(milliseconds to wait=u32 10) -> ()  [unwired: 1 out]
        }
        frame #1 {
          # "Set to shot location"
          n129 = while {
            stop <- TRUE stop-if-true
            n130 = call "Set Shooter Config.vi"("POV Joystick Input"=270) -> ()  [unwired: 3 in]
          }
          n131 = Wait (ms)(milliseconds to wait=u32 10) -> ()  [unwired: 1 out]
        }
        frame #2 {
          # "Intake Pivot out"
          n132 = call <vilib>:"WPI_SolenoidRefNum Registry Get.vi"("refnum name"="Intake Pivot") -> ("error out"=w422:errorcluster, "SolenoidDevRef"=w421:T12)  [unwired: 9 in]
          n133 = call-poly <vilib>:"WPI_SolenoidSet.vi"("error in (no error)"=w422, "Value"=WPI_SolenoidValue."Reverse", "SolenoidDevRef"=w421) -> ()  [unwired: 7 in, 2 out]
        }
        frame #3 {
          w424 = 0.7 ("Output")
          n134 = call <vilib>:"WPI_MotorControlRefNum Registry Get.vi"("refnum name"="Intake") -> ("MotorControlDevRef"=w427:T5)  [unwired: 9 in, 1 out]
          n135 = call <vilib>:"WPI_MotorControlRefNum Registry Get.vi"("refnum name"="Singulator") -> ("MotorControlDevRef"=w428:T5)  [unwired: 9 in, 1 out]
          n136 = Wait (ms)(milliseconds to wait=u32 1000) -> ()  [unwired: 1 out]
          n137 = call <vilib>:"WPI_MotorControlSetOutput.vi"("Output"=w424, "MotorControlDevRef"=w428) -> ("MotorControlDevRef"=w426:T5)  [unwired: 7 in, 2 out]
          n138 = call <vilib>:"WPI_MotorControlSetOutput.vi"("Output"=w424, "MotorControlDevRef"=w427) -> ("MotorControlDevRef"=w425:T5)  [unwired: 7 in, 2 out]
        }
        frame #4 {
          # "Drive to HP"
          n139 = Wait (ms)(milliseconds to wait=u32 2800) -> ()  [unwired: 1 out]
          n140 = call <vilib>:"WPI_RobotDriveRefNum Registry Get.vi"("refnum name"="6MRobotDrive") -> ("error out"=w442:errorcluster, "RobotDriveDevRef"=w441:T4)  [unwired: 1 in, 8 out]
          n141 = call <vilib>:"WPI_RobotDriveArcadeDrive_Standard(NoSaturation).vi"("Y axis value"=0.0, "X axis value"=0.7, "RobotDriveDevRef"=w441) -> ()  [unwired: 1 in, 8 out]
          n142 = call <vilib>:"WPI_RobotDriveSafetyConfig.vi"("error in (no error)"=w442, "mode"=WPI_SafetyOutputConfigMenu."Disable", "RobotDriveDevRef"=w441) -> ("error out"=w439:errorcluster, "RobotDriveDevRef"=w433:T4)  [unwired: 7 in]
        }
        frame #5 {
          w448 = 0.0 ("Output")
          # "Drive to fender intake off"
          n143 = Wait (ms)(milliseconds to wait=u32 200) -> ()  [unwired: 1 out]
          n144 = call <vilib>:"WPI_MotorControlSetOutput.vi"("Output"=w448, "MotorControlDevRef"=w449) -> ()  [unwired: 7 in, 3 out]
          n145 = call <vilib>:"WPI_MotorControlSetOutput.vi"("Output"=w448, "MotorControlDevRef"=w450) -> ()  [unwired: 7 in, 3 out]
        }
        frame #6 {
          n146 = call <vilib>:"WPI_RobotDriveArcadeDrive_Standard(NoSaturation).vi"("error in (no error)"=w454, "Y axis value"=0.0, "X axis value"=0.0, "RobotDriveDevRef"=w455) -> ()  [unwired: 8 out]
        }
        frame #7 {
          # "Turn on Shooter"
          n147 = global read "Global Shooter Speed.vi" "Shooter Speed Target"() -> (w466:dbl)
          n148 = global read "Global Shooter Speed.vi" "Accelerator Speed Target"() -> (w464:dbl)
          n149 = call <vilib>:"Spark MAX Set Output Advanced.vi"("Control Mode"=Spark_MAX_Control_Type."Velocity", "Setpoint"=w466, "MotorControlDevRef"=w461) -> ("MotorControlDevRef"=w460:T5)  [unwired: 7 in, 1 out]
          n150 = call <vilib>:"Spark MAX Set Output Advanced.vi"("Control Mode"=Spark_MAX_Control_Type."Velocity", "Setpoint"=w464, "MotorControlDevRef"=w463) -> ("MotorControlDevRef"=w462:T5)  [unwired: 7 in, 1 out]
        }
        frame #8 {
          n151 = Wait (ms)(milliseconds to wait=u32 3000) -> ()  [unwired: 1 out]
        }
        frame #9 {
          # "Feed"
          n152 = Wait (ms)(milliseconds to wait=u32 2000) -> ()  [unwired: 1 out]
          n153 = call "Feed to Shooter.vi"("Feed Input"=0.3) -> ()  [unwired: 11 in]
        }
        frame #10 {
          # "Turn Off"
          n154 = call <vilib>:"WPI_RobotDriveArcadeDrive_Standard(NoSaturation).vi"("error in (no error)"=w484, "Y axis value"=0.0, "X axis value"=0.0, "RobotDriveDevRef"=w485) -> ()  [unwired: 8 out]
          n155 = call "Feed to Shooter.vi"("Feed Input"=0.0) -> ()  [unwired: 11 in]
          n156 = Wait (ms)(milliseconds to wait=u32 1000) -> ()  [unwired: 1 out]
        }
        frame #11 {
          n157 = call <vilib>:"WPI_MotorControlSetOutput.vi"("Output"=0.0, "MotorControlDevRef"=w489) -> ()  [unwired: 7 in, 3 out]
          n158 = call <vilib>:"WPI_MotorControlSetOutput.vi"("Output"=0.0, "MotorControlDevRef"=w491) -> ()  [unwired: 7 in, 3 out]
        }
      }
    }
    frame "Drive Shoot Two Fast" {
      n159 = flat-sequence {
        tunnel: w535 -> [w540]
        tunnel: w537 -> [w541]
        tunnel: [w541] -> w532
        tunnel: [w540] -> w531
        tunnel: [w543] -> w538
        tunnel: [w542] -> w536
        tunnel: w532 -> [w543]
        tunnel: w531 -> [w542]
        tunnel: w538 -> [w548]
        tunnel: w536 -> [w547]
        tunnel: [w548] -> w526
        tunnel: [w547] -> w523
        tunnel: [w562] -> w527
        tunnel: w526 -> [w562]
        tunnel: [w561] -> w524
        tunnel: w523 -> [w561]
        tunnel: [w556] -> w517
        tunnel: [w555] -> w515
        tunnel: [w569] -> w530
        tunnel: [w568] -> w529
        tunnel: [w566] -> w528
        tunnel: w527 -> [w566]
        tunnel: [w565] -> w525
        tunnel: w524 -> [w565]
        tunnel: [w564] -> w518
        tunnel: w517 -> [w564]
        tunnel: [w563] -> w516
        tunnel: w515 -> [w563]
        tunnel: w530 -> [w581]
        tunnel: [w581] -> w502
        tunnel: w529 -> [w584]
        tunnel: [w584] -> w500
        tunnel: [w578] -> w498
        tunnel: [w579] -> w496
        tunnel: w528 -> [w579]
        tunnel: w525 -> [w578]
        tunnel: w518 -> [w576]
        tunnel: w516 -> [w577]
        tunnel: [w577] -> w494
        tunnel: [w576] -> w493
        tunnel: w502 -> [w592]
        tunnel: [w592] -> w501
        tunnel: w500 -> [w591]
        tunnel: [w591] -> w499
        tunnel: w498 -> [w590]
        tunnel: [w590] -> w497
        tunnel: w496 -> [w589]
        tunnel: [w589] -> w495
        tunnel: w494 -> [w588]
        tunnel: w493 -> [w587]
        tunnel: w501 -> [w594]
        tunnel: [w594] -> w506
        tunnel: w499 -> [w593]
        tunnel: [w593] -> w505
        tunnel: w497 -> [w598]
        tunnel: [w598] -> w504
        tunnel: w495 -> [w597]
        tunnel: [w597] -> w503
        tunnel: w506 -> [w608]
        tunnel: [w608] -> w514
        tunnel: w505 -> [w607]
        tunnel: [w607] -> w512
        tunnel: [w599] -> w510
        tunnel: w504 -> [w602]
        tunnel: [w601] -> w508
        tunnel: w503 -> [w600]
        tunnel: w514 -> [w613]
        tunnel: [w613] -> w513
        tunnel: w512 -> [w612]
        tunnel: [w612] -> w511
        tunnel: w510 -> [w611]
        tunnel: [w611] -> w509
        tunnel: w508 -> [w610]
        tunnel: [w610] -> w507
        tunnel: w513 -> [w619]
        tunnel: [w619] -> w522
        tunnel: w511 -> [w618]
        tunnel: [w618] -> w521
        tunnel: w509 -> [w617]
        tunnel: [w617] -> w520
        tunnel: w507 -> [w616]
        tunnel: [w616] -> w519
        tunnel: w522 -> [w624]
        tunnel: w521 -> [w623]
        tunnel: w520 -> [w620]
        tunnel: w519 -> [w621]
        tunnel: [w621] -> w534
        tunnel: [w620] -> w533
        tunnel: w534 -> [w630]
        tunnel: w533 -> [w628]
        frame #0 {
          n160 = Wait (ms)(milliseconds to wait=u32 10) -> ()  [unwired: 1 out]
        }
        frame #1 {
          # "Set to shot location"
          n161 = while {
            stop <- TRUE stop-if-true
            n162 = call "Set Shooter Config.vi"("POV Joystick Input"=270) -> ()  [unwired: 3 in]
          }
          n163 = Wait (ms)(milliseconds to wait=u32 10) -> ()  [unwired: 1 out]
        }
        frame #2 {
          # "Intake Pivot out"
          n164 = call <vilib>:"WPI_SolenoidRefNum Registry Get.vi"("refnum name"="Intake Pivot") -> ("error out"=w552:errorcluster, "SolenoidDevRef"=w551:T12)  [unwired: 9 in]
          n165 = call-poly <vilib>:"WPI_SolenoidSet.vi"("error in (no error)"=w552, "Value"=WPI_SolenoidValue."Reverse", "SolenoidDevRef"=w551) -> ()  [unwired: 7 in, 2 out]
        }
        frame #3 {
          w554 = 0.7 ("Output")
          n166 = call <vilib>:"WPI_MotorControlRefNum Registry Get.vi"("refnum name"="Intake") -> ("MotorControlDevRef"=w557:T5)  [unwired: 9 in, 1 out]
          n167 = call <vilib>:"WPI_MotorControlRefNum Registry Get.vi"("refnum name"="Singulator") -> ("MotorControlDevRef"=w558:T5)  [unwired: 9 in, 1 out]
          n168 = Wait (ms)(milliseconds to wait=u32 10) -> ()  [unwired: 1 out]
          n169 = call <vilib>:"WPI_MotorControlSetOutput.vi"("Output"=w554, "MotorControlDevRef"=w558) -> ("MotorControlDevRef"=w556:T5)  [unwired: 7 in, 2 out]
          n170 = call <vilib>:"WPI_MotorControlSetOutput.vi"("Output"=w554, "MotorControlDevRef"=w557) -> ("MotorControlDevRef"=w555:T5)  [unwired: 7 in, 2 out]
        }
        frame #4 {
          # "Drive away from Hub"
          n171 = Wait (ms)(milliseconds to wait=u32 1000) -> ()  [unwired: 1 out]
          n172 = call <vilib>:"WPI_RobotDriveRefNum Registry Get.vi"("refnum name"="6MRobotDrive") -> ("error out"=w572:errorcluster, "RobotDriveDevRef"=w571:T4)  [unwired: 1 in, 8 out]
          n173 = call <vilib>:"WPI_RobotDriveArcadeDrive_Standard(NoSaturation).vi"("Y axis value"=0.0, "X axis value"=-0.7, "RobotDriveDevRef"=w571) -> ()  [unwired: 1 in, 8 out]
          n174 = call <vilib>:"WPI_RobotDriveSafetyConfig.vi"("error in (no error)"=w572, "mode"=WPI_SafetyOutputConfigMenu."Disable", "RobotDriveDevRef"=w571) -> ("error out"=w568:errorcluster, "RobotDriveDevRef"=w569:T4)  [unwired: 7 in]
        }
        frame #5 {
          # "Drive to Fender and intake"
          n175 = Wait (ms)(milliseconds to wait=u32 800) -> ()  [unwired: 1 out]
          n176 = call <vilib>:"WPI_RobotDriveArcadeDrive_Standard(NoSaturation).vi"("Y axis value"=0.0, "X axis value"=0.7, "RobotDriveDevRef"=w581) -> ()  [unwired: 1 in, 8 out]
        }
        frame #6 {
          w586 = 0.0 ("Output")
          # "Drive to fender intake off"
          n177 = Wait (ms)(milliseconds to wait=u32 200) -> ()  [unwired: 1 out]
          n178 = call <vilib>:"WPI_MotorControlSetOutput.vi"("Output"=w586, "MotorControlDevRef"=w587) -> ()  [unwired: 7 in, 3 out]
          n179 = call <vilib>:"WPI_MotorControlSetOutput.vi"("Output"=w586, "MotorControlDevRef"=w588) -> ()  [unwired: 7 in, 3 out]
        }
        frame #7 {
          n180 = call <vilib>:"WPI_RobotDriveArcadeDrive_Standard(NoSaturation).vi"("error in (no error)"=w593, "Y axis value"=0.0, "X axis value"=0.0, "RobotDriveDevRef"=w594) -> ()  [unwired: 8 out]
        }
        frame #8 {
          # "Turn on Shooter"
          n181 = global read "Global Shooter Speed.vi" "Shooter Speed Target"() -> (w605:dbl)
          n182 = global read "Global Shooter Speed.vi" "Accelerator Speed Target"() -> (w603:dbl)
          n183 = call <vilib>:"Spark MAX Set Output Advanced.vi"("Control Mode"=Spark_MAX_Control_Type."Velocity", "Setpoint"=w605, "MotorControlDevRef"=w600) -> ("MotorControlDevRef"=w599:T5)  [unwired: 7 in, 1 out]
          n184 = call <vilib>:"Spark MAX Set Output Advanced.vi"("Control Mode"=Spark_MAX_Control_Type."Velocity", "Setpoint"=w603, "MotorControlDevRef"=w602) -> ("MotorControlDevRef"=w601:T5)  [unwired: 7 in, 1 out]
        }
        frame #9 {
          n185 = Wait (ms)(milliseconds to wait=u32 1500) -> ()  [unwired: 1 out]
        }
        frame #10 {
          # "Feed"
          n186 = Wait (ms)(milliseconds to wait=u32 2000) -> ()  [unwired: 1 out]
          n187 = call "Feed to Shooter.vi"("Feed Input"=0.3) -> ()  [unwired: 11 in]
        }
        frame #11 {
          # "Turn Off"
          n188 = call <vilib>:"WPI_RobotDriveArcadeDrive_Standard(NoSaturation).vi"("error in (no error)"=w623, "Y axis value"=0.0, "X axis value"=0.0, "RobotDriveDevRef"=w624) -> ()  [unwired: 8 out]
          n189 = call "Feed to Shooter.vi"("Feed Input"=0.0) -> ()  [unwired: 11 in]
          n190 = Wait (ms)(milliseconds to wait=u32 1000) -> ()  [unwired: 1 out]
        }
        frame #12 {
          n191 = call <vilib>:"WPI_MotorControlSetOutput.vi"("Output"=0.0, "MotorControlDevRef"=w628) -> ()  [unwired: 7 in, 3 out]
          n192 = call <vilib>:"WPI_MotorControlSetOutput.vi"("Output"=0.0, "MotorControlDevRef"=w630) -> ()  [unwired: 7 in, 3 out]
        }
      }
    }
    frame "Drive Shoot Drive Pickup" {
      n193 = flat-sequence {
        tunnel: w710 -> [w715]
        tunnel: w712 -> [w716]
        tunnel: [w716] -> w707
        tunnel: [w715] -> w706
        tunnel: [w718] -> w713
        tunnel: [w717] -> w711
        tunnel: w707 -> [w718]
        tunnel: w706 -> [w717]
        tunnel: w713 -> [w723]
        tunnel: w711 -> [w722]
        tunnel: [w723] -> w701
        tunnel: [w722] -> w698
        tunnel: [w737] -> w702
        tunnel: w701 -> [w737]
        tunnel: [w736] -> w699
        tunnel: w698 -> [w736]
        tunnel: [w731] -> w696
        tunnel: [w730] -> w694
        tunnel: [w744] -> w705
        tunnel: [w743] -> w704
        tunnel: [w741] -> w703
        tunnel: w702 -> [w741]
        tunnel: [w740] -> w700
        tunnel: w699 -> [w740]
        tunnel: [w739] -> w697
        tunnel: w696 -> [w739]
        tunnel: [w738] -> w695
        tunnel: w694 -> [w738]
        tunnel: w705 -> [w756]
        tunnel: [w756] -> w681
        tunnel: w704 -> [w759]
        tunnel: [w759] -> w679
        tunnel: [w753] -> w677
        tunnel: [w754] -> w675
        tunnel: w703 -> [w754]
        tunnel: w700 -> [w753]
        tunnel: w697 -> [w751]
        tunnel: w695 -> [w752]
        tunnel: [w752] -> w673
        tunnel: [w751] -> w672
        tunnel: w681 -> [w769]
        tunnel: [w769] -> w680
        tunnel: w679 -> [w768]
        tunnel: [w768] -> w678
        tunnel: w677 -> [w767]
        tunnel: [w767] -> w676
        tunnel: w675 -> [w766]
        tunnel: [w766] -> w674
        tunnel: w673 -> [w765]
        tunnel: w672 -> [w764]
        tunnel: [w761] -> w652
        tunnel: [w760] -> w645
        tunnel: w680 -> [w773]
        tunnel: [w773] -> w685
        tunnel: w678 -> [w772]
        tunnel: [w772] -> w684
        tunnel: w676 -> [w777]
        tunnel: [w777] -> w683
        tunnel: w674 -> [w776]
        tunnel: [w776] -> w682
        tunnel: [w771] -> w653
        tunnel: w652 -> [w771]
        tunnel: [w770] -> w646
        tunnel: w645 -> [w770]
        tunnel: w685 -> [w789]
        tunnel: [w789] -> w693
        tunnel: w684 -> [w788]
        tunnel: [w788] -> w691
        tunnel: [w780] -> w689
        tunnel: w683 -> [w783]
        tunnel: [w782] -> w687
        tunnel: w682 -> [w781]
        tunnel: [w779] -> w654
        tunnel: w653 -> [w779]
        tunnel: [w778] -> w647
        tunnel: w646 -> [w778]
        tunnel: w693 -> [w796]
        tunnel: [w796] -> w692
        tunnel: w691 -> [w795]
        tunnel: [w795] -> w690
        tunnel: w689 -> [w794]
        tunnel: [w794] -> w688
        tunnel: w687 -> [w793]
        tunnel: [w793] -> w686
        tunnel: [w791] -> w655
        tunnel: w654 -> [w791]
        tunnel: [w790] -> w648
        tunnel: w647 -> [w790]
        tunnel: w692 -> [w804]
        tunnel: [w804] -> w671
        tunnel: w690 -> [w803]
        tunnel: [w803] -> w669
        tunnel: w688 -> [w802]
        tunnel: [w802] -> w667
        tunnel: w686 -> [w801]
        tunnel: [w801] -> w665
        tunnel: [w798] -> w656
        tunnel: w655 -> [w798]
        tunnel: [w797] -> w649
        tunnel: w648 -> [w797]
        tunnel: w671 -> [w814]
        tunnel: [w814] -> w670
        tunnel: w669 -> [w813]
        tunnel: [w813] -> w668
        tunnel: w667 -> [w812]
        tunnel: [w812] -> w666
        tunnel: w665 -> [w811]
        tunnel: [w811] -> w664
        tunnel: [w810] -> w663
        tunnel: [w806] -> w657
        tunnel: w656 -> [w806]
        tunnel: [w805] -> w650
        tunnel: w649 -> [w805]
        tunnel: w670 -> [w821]
        tunnel: w668 -> [w820]
        tunnel: [w819] -> w662
        tunnel: w666 -> [w823]
        tunnel: [w823] -> w661
        tunnel: w664 -> [w822]
        tunnel: [w822] -> w660
        tunnel: w663 -> [w818]
        tunnel: [w817] -> w659
        tunnel: [w816] -> w658
        tunnel: w657 -> [w816]
        tunnel: [w815] -> w651
        tunnel: w650 -> [w815]
        tunnel: [w845] -> w644
        tunnel: w662 -> [w842]
        tunnel: [w841] -> w642
        tunnel: w661 -> [w837]
        tunnel: w660 -> [w847]
        tunnel: [w847] -> w639
        tunnel: w659 -> [w846]
        tunnel: w658 -> [w838]
        tunnel: w651 -> [w839]
        tunnel: [w838] -> w637
        tunnel: [w837] -> w636
        tunnel: [w836] -> w633
        tunnel: [w835] -> w632
        tunnel: w644 -> [w854]
        tunnel: [w854] -> w643
        tunnel: w642 -> [w853]
        tunnel: [w853] -> w641
        tunnel: [w852] -> w640
        tunnel: w639 -> [w851]
        tunnel: [w851] -> w638
        tunnel: w637 -> [_]
        tunnel: w636 -> [w852]
        tunnel: [w849] -> w635
        tunnel: [w848] -> w634
        tunnel: w633 -> [w849]
        tunnel: w632 -> [w848]
        tunnel: w643 -> [w861]
        tunnel: w641 -> [w860]
        tunnel: w640 -> [w858]
        tunnel: w638 -> [w859]
        tunnel: [w859] -> w709
        tunnel: [w858] -> w708
        tunnel: w635 -> [w857]
        tunnel: w634 -> [w856]
        tunnel: w709 -> [w867]
        tunnel: w708 -> [w865]
        frame #0 {
          n194 = Wait (ms)(milliseconds to wait=u32 10) -> ()  [unwired: 1 out]
        }
        frame #1 {
          # "Set to shot location"
          n195 = while {
            stop <- TRUE stop-if-true
            n196 = call "Set Shooter Config.vi"("POV Joystick Input"=270) -> ()  [unwired: 3 in]
          }
          n197 = Wait (ms)(milliseconds to wait=u32 10) -> ()  [unwired: 1 out]
        }
        frame #2 {
          # "Intake Pivot out"
          n198 = call <vilib>:"WPI_SolenoidRefNum Registry Get.vi"("refnum name"="Intake Pivot") -> ("error out"=w727:errorcluster, "SolenoidDevRef"=w726:T12)  [unwired: 9 in]
          n199 = call-poly <vilib>:"WPI_SolenoidSet.vi"("error in (no error)"=w727, "Value"=WPI_SolenoidValue."Reverse", "SolenoidDevRef"=w726) -> ()  [unwired: 7 in, 2 out]
        }
        frame #3 {
          w729 = 0.7 ("Output")
          n200 = call <vilib>:"WPI_MotorControlRefNum Registry Get.vi"("refnum name"="Intake") -> ("MotorControlDevRef"=w732:T5)  [unwired: 9 in, 1 out]
          n201 = call <vilib>:"WPI_MotorControlRefNum Registry Get.vi"("refnum name"="Singulator") -> ("MotorControlDevRef"=w733:T5)  [unwired: 9 in, 1 out]
          n202 = Wait (ms)(milliseconds to wait=u32 10) -> ()  [unwired: 1 out]
          n203 = call <vilib>:"WPI_MotorControlSetOutput.vi"("Output"=w729, "MotorControlDevRef"=w733) -> ("MotorControlDevRef"=w731:T5)  [unwired: 7 in, 2 out]
          n204 = call <vilib>:"WPI_MotorControlSetOutput.vi"("Output"=w729, "MotorControlDevRef"=w732) -> ("MotorControlDevRef"=w730:T5)  [unwired: 7 in, 2 out]
        }
        frame #4 {
          # "Drive away from Hub"
          n205 = Wait (ms)(milliseconds to wait=u32 1000) -> ()  [unwired: 1 out]
          n206 = call <vilib>:"WPI_RobotDriveRefNum Registry Get.vi"("refnum name"="6MRobotDrive") -> ("error out"=w747:errorcluster, "RobotDriveDevRef"=w746:T4)  [unwired: 1 in, 8 out]
          n207 = call <vilib>:"WPI_RobotDriveArcadeDrive_Standard(NoSaturation).vi"("Y axis value"=0.0, "X axis value"=-0.7, "RobotDriveDevRef"=w746) -> ()  [unwired: 1 in, 8 out]
          n208 = call <vilib>:"WPI_RobotDriveSafetyConfig.vi"("error in (no error)"=w747, "mode"=WPI_SafetyOutputConfigMenu."Disable", "RobotDriveDevRef"=w746) -> ("error out"=w743:errorcluster, "RobotDriveDevRef"=w744:T4)  [unwired: 7 in]
        }
        frame #5 {
          # "Drive to Fender and intake"
          n209 = Wait (ms)(milliseconds to wait=u32 800) -> ()  [unwired: 1 out]
          n210 = call <vilib>:"WPI_RobotDriveArcadeDrive_Standard(NoSaturation).vi"("Y axis value"=0.0, "X axis value"=0.7, "RobotDriveDevRef"=w756) -> ()  [unwired: 1 in, 8 out]
        }
        frame #6 {
          w763 = 0.0 ("Output")
          # "Drive to fender intake off"
          n211 = Wait (ms)(milliseconds to wait=u32 200) -> ()  [unwired: 1 out]
          n212 = call <vilib>:"WPI_MotorControlSetOutput.vi"("Output"=w763, "MotorControlDevRef"=w764) -> ("MotorControlDevRef"=w761:T5)  [unwired: 7 in, 2 out]
          n213 = call <vilib>:"WPI_MotorControlSetOutput.vi"("Output"=w763, "MotorControlDevRef"=w765) -> ("MotorControlDevRef"=w760:T5)  [unwired: 7 in, 2 out]
        }
        frame #7 {
          n214 = call <vilib>:"WPI_RobotDriveArcadeDrive_Standard(NoSaturation).vi"("error in (no error)"=w772, "Y axis value"=0.0, "X axis value"=0.0, "RobotDriveDevRef"=w773) -> ()  [unwired: 8 out]
        }
        frame #8 {
          # "Turn on Shooter"
          n215 = global read "Global Shooter Speed.vi" "Shooter Speed Target"() -> (w786:dbl)
          n216 = global read "Global Shooter Speed.vi" "Accelerator Speed Target"() -> (w784:dbl)
          n217 = call <vilib>:"Spark MAX Set Output Advanced.vi"("Control Mode"=Spark_MAX_Control_Type."Velocity", "Setpoint"=w786, "MotorControlDevRef"=w781) -> ("MotorControlDevRef"=w780:T5)  [unwired: 7 in, 1 out]
          n218 = call <vilib>:"Spark MAX Set Output Advanced.vi"("Control Mode"=Spark_MAX_Control_Type."Velocity", "Setpoint"=w784, "MotorControlDevRef"=w783) -> ("MotorControlDevRef"=w782:T5)  [unwired: 7 in, 1 out]
        }
        frame #9 {
          n219 = Wait (ms)(milliseconds to wait=u32 1000) -> ()  [unwired: 1 out]
        }
        frame #10 {
          # "Feed"
          n220 = Wait (ms)(milliseconds to wait=u32 2000) -> ()  [unwired: 1 out]
          n221 = call "Feed to Shooter.vi"("Feed Input"=0.3) -> ()  [unwired: 11 in]
        }
        frame #11 {
          n222 = call <vilib>:"WPI_GyroRefNum Registry Get.vi"("refnum name"="AD Gyro") -> ("GyroDevRef"=w809:T14)  [unwired: 9 in, 1 out]
          n223 = call "Feed to Shooter.vi"("Feed Input"=0.0) -> ()  [unwired: 11 in]
          n224 = call <vilib>:"WPI_GyroReset.vi"("GyroDevRef"=w809) -> ("GyroDevRef"=w810:T14)  [unwired: 9 in, 1 out]
        }
        frame #12 {
          n225 = while {
            shift-right: [w832] -> w817
            shift-left: w821 -> [w833]
            shift-right: [w828] -> w819
            shift-left: w820 -> [w829]
            tunnel: w818 -> [w827]
            stop <- w824 stop-if-true
            n226 = call <vilib>:"WPI_RobotDriveArcadeDrive_Standard(NoSaturation).vi"("error in (no error)"=w829, "Y axis value"=0.48, "X axis value"=0.0, "RobotDriveDevRef"=w833) -> ("error out"=w828:errorcluster, "RobotDriveDevRef"=w832:T4)  [unwired: 6 out]
            n227 = call <vilib>:"WPI_GyroGetAngle.vi"("GyroDevRef"=w827) -> ("Angle"=w825:dbl)  [unwired: 6 in, 4 out]
            n228 = Less Or Equal?(x=w825, y=-55.0) -> (x <= y?=w824:bool)
          }
        }
        frame #13 {
          w834 = 0.7 ("Output")
          n229 = call <vilib>:"WPI_MotorControlSetOutput.vi"("Output"=w834, "MotorControlDevRef"=w839) -> ("MotorControlDevRef"=w835:T5)  [unwired: 7 in, 2 out]
          n230 = Wait (ms)(milliseconds to wait=u32 600) -> ()  [unwired: 1 out]
          n231 = call <vilib>:"WPI_RobotDriveArcadeDrive_Standard(NoSaturation).vi"("error in (no error)"=w842, "Y axis value"=0.0, "X axis value"=-0.7, "RobotDriveDevRef"=w846) -> ("error out"=w841:errorcluster, "RobotDriveDevRef"=w845:T4)  [unwired: 6 out]
          n232 = call <vilib>:"WPI_MotorControlSetOutput.vi"("Output"=w834, "MotorControlDevRef"=w838) -> ("MotorControlDevRef"=w836:T5)  [unwired: 7 in, 2 out]
        }
        frame #14 {
          n233 = Wait (ms)(milliseconds to wait=u32 1000) -> ()  [unwired: 1 out]
        }
        frame #15 {
          w855 = 0.0 ("Output")
          # "Turn Off"
          n234 = call <vilib>:"WPI_MotorControlSetOutput.vi"("Output"=w855, "MotorControlDevRef"=w857) -> ()  [unwired: 7 in, 3 out]
          n235 = call <vilib>:"WPI_MotorControlSetOutput.vi"("Output"=w855, "MotorControlDevRef"=w856) -> ()  [unwired: 7 in, 3 out]
          n236 = call <vilib>:"WPI_RobotDriveArcadeDrive_Standard(NoSaturation).vi"("error in (no error)"=w860, "Y axis value"=0.0, "X axis value"=0.0, "RobotDriveDevRef"=w861) -> ()  [unwired: 8 out]
          n237 = Wait (ms)(milliseconds to wait=u32 1000) -> ()  [unwired: 1 out]
        }
        frame #16 {
          n238 = call <vilib>:"WPI_MotorControlSetOutput.vi"("Output"=0.0, "MotorControlDevRef"=w865) -> ()  [unwired: 7 in, 3 out]
          n239 = call <vilib>:"WPI_MotorControlSetOutput.vi"("Output"=0.0, "MotorControlDevRef"=w867) -> ()  [unwired: 7 in, 3 out]
        }
      }
    }
    frame "Right Multiball" {
      n240 = flat-sequence {
        tunnel: w999 -> [w1006]
        tunnel: w1001 -> [w1007]
        tunnel: [w1007] -> w996
        tunnel: [w1006] -> w995
        tunnel: [w1009] -> w1002
        tunnel: [w1008] -> w1000
        tunnel: w996 -> [w1009]
        tunnel: w995 -> [w1008]
        tunnel: w1002 -> [w1014]
        tunnel: w1000 -> [w1013]
        tunnel: [w1014] -> w990
        tunnel: [w1013] -> w987
        tunnel: [w1028] -> w991
        tunnel: w990 -> [w1028]
        tunnel: [w1027] -> w988
        tunnel: w987 -> [w1027]
        tunnel: [w1022] -> w985
        tunnel: [w1021] -> w983
        tunnel: [w1035] -> w994
        tunnel: [w1034] -> w993
        tunnel: [w1032] -> w992
        tunnel: w991 -> [w1032]
        tunnel: [w1031] -> w989
        tunnel: w988 -> [w1031]
        tunnel: [w1030] -> w986
        tunnel: w985 -> [w1030]
        tunnel: [w1029] -> w984
        tunnel: w983 -> [w1029]
        tunnel: w994 -> [w1047]
        tunnel: [w1047] -> w970
        tunnel: w993 -> [w1050]
        tunnel: [w1050] -> w968
        tunnel: [w1044] -> w966
        tunnel: [w1045] -> w964
        tunnel: w992 -> [w1045]
        tunnel: w989 -> [w1044]
        tunnel: w986 -> [w1042]
        tunnel: w984 -> [w1043]
        tunnel: [w1043] -> w962
        tunnel: [w1042] -> w961
        tunnel: w970 -> [w1060]
        tunnel: [w1060] -> w969
        tunnel: w968 -> [w1059]
        tunnel: [w1059] -> w967
        tunnel: w966 -> [w1058]
        tunnel: [w1058] -> w965
        tunnel: w964 -> [w1057]
        tunnel: [w1057] -> w963
        tunnel: w962 -> [w1056]
        tunnel: w961 -> [w1055]
        tunnel: [w1052] -> w945
        tunnel: [w1051] -> w938
        tunnel: w969 -> [w1064]
        tunnel: [w1064] -> w974
        tunnel: w967 -> [w1063]
        tunnel: [w1063] -> w973
        tunnel: w965 -> [w1068]
        tunnel: [w1068] -> w972
        tunnel: w963 -> [w1067]
        tunnel: [w1067] -> w971
        tunnel: [w1062] -> w946
        tunnel: w945 -> [w1062]
        tunnel: [w1061] -> w939
        tunnel: w938 -> [w1061]
        tunnel: w974 -> [w1081]
        tunnel: [w1081] -> w982
        tunnel: w973 -> [w1080]
        tunnel: [w1080] -> w980
        tunnel: [w1072] -> w978
        tunnel: w972 -> [w1075]
        tunnel: [w1074] -> w976
        tunnel: w971 -> [w1073]
        tunnel: [w1071] -> w947
        tunnel: w946 -> [w1071]
        tunnel: [w1070] -> w940
        tunnel: w939 -> [w1070]
        tunnel: w982 -> [w1087]
        tunnel: [w1087] -> w981
        tunnel: w980 -> [w1086]
        tunnel: [w1086] -> w979
        tunnel: w978 -> [w1085]
        tunnel: [w1085] -> w977
        tunnel: w976 -> [w1084]
        tunnel: [w1084] -> w975
        tunnel: [w1083] -> w948
        tunnel: w947 -> [w1083]
        tunnel: [w1082] -> w941
        tunnel: w940 -> [w1082]
        tunnel: w981 -> [w1095]
        tunnel: [w1095] -> w960
        tunnel: w979 -> [w1094]
        tunnel: [w1094] -> w958
        tunnel: w977 -> [w1093]
        tunnel: [w1093] -> w956
        tunnel: w975 -> [w1092]
        tunnel: [w1092] -> w954
        tunnel: [w1089] -> w949
        tunnel: w948 -> [w1089]
        tunnel: [w1088] -> w942
        tunnel: w941 -> [w1088]
        tunnel: w960 -> [w1103]
        tunnel: [w1103] -> w959
        tunnel: w958 -> [w1102]
        tunnel: [w1102] -> w957
        tunnel: w956 -> [w1101]
        tunnel: [w1101] -> w955
        tunnel: w954 -> [w1100]
        tunnel: [w1100] -> w953
        tunnel: [w1098] -> w950
        tunnel: w949 -> [w1098]
        tunnel: [w1097] -> w943
        tunnel: w942 -> [w1097]
        tunnel: w959 -> [w1115]
        tunnel: w957 -> [w1114]
        tunnel: [w1113] -> w952
        tunnel: w955 -> [w1107]
        tunnel: w953 -> [w1110]
        tunnel: [w1112] -> w951
        tunnel: w950 -> [w1104]
        tunnel: [w1111] -> w944
        tunnel: w943 -> [w1111]
        tunnel: [w1109] -> w910
        tunnel: [w1106] -> w909
        tunnel: [w1104] -> w870
        tunnel: [w1131] -> w937
        tunnel: w952 -> [w1128]
        tunnel: [w1127] -> w936
        tunnel: [w1133] -> w935
        tunnel: w951 -> [w1132]
        tunnel: w944 -> [w1122]
        tunnel: [w1125] -> w934
        tunnel: w910 -> [w1133]
        tunnel: w909 -> [w1125]
        tunnel: [w1124] -> w871
        tunnel: w870 -> [w1123]
        tunnel: [w1121] -> w869
        tunnel: w937 -> [w1142]
        tunnel: [w1141] -> w916
        tunnel: w936 -> [w1138]
        tunnel: [w1137] -> w915
        tunnel: w935 -> [w1144]
        tunnel: [w1144] -> w914
        tunnel: w934 -> [w1143]
        tunnel: [w1143] -> w913
        tunnel: [w1134] -> w912
        tunnel: [w1135] -> w911
        tunnel: w871 -> [w1135]
        tunnel: w869 -> [w1134]
        tunnel: w916 -> [w1150]
        tunnel: [w1150] -> w883
        tunnel: w915 -> [w1149]
        tunnel: [w1149] -> w881
        tunnel: w914 -> [w1148]
        tunnel: [w1148] -> w879
        tunnel: w913 -> [w1147]
        tunnel: [w1147] -> w877
        tunnel: w912 -> [w1146]
        tunnel: [w1146] -> w875
        tunnel: w911 -> [w1145]
        tunnel: [w1145] -> w873
        tunnel: w883 -> [w1162]
        tunnel: [w1162] -> w882
        tunnel: w881 -> [w1161]
        tunnel: [w1161] -> w880
        tunnel: w879 -> [w1160]
        tunnel: [w1160] -> w878
        tunnel: w877 -> [w1159]
        tunnel: [w1159] -> w876
        tunnel: w875 -> [w1154]
        tunnel: [w1156] -> w874
        tunnel: w873 -> [w1155]
        tunnel: [w1157] -> w872
        tunnel: w882 -> [w1177]
        tunnel: [w1177] -> w922
        tunnel: w880 -> [w1176]
        tunnel: [w1176] -> w921
        tunnel: w878 -> [w1167]
        tunnel: [w1166] -> w920
        tunnel: w876 -> [w1169]
        tunnel: [w1168] -> w919
        tunnel: w874 -> [w1175]
        tunnel: [w1175] -> w918
        tunnel: w872 -> [w1174]
        tunnel: [w1174] -> w917
        tunnel: w922 -> [w1185]
        tunnel: [w1185] -> w908
        tunnel: w921 -> [w1184]
        tunnel: [w1184] -> w906
        tunnel: w920 -> [w1183]
        tunnel: [w1183] -> w904
        tunnel: w919 -> [w1182]
        tunnel: [w1182] -> w902
        tunnel: w918 -> [w1181]
        tunnel: [w1181] -> w900
        tunnel: w917 -> [w1180]
        tunnel: [w1180] -> w898
        tunnel: w908 -> [w1192]
        tunnel: [w1192] -> w907
        tunnel: w906 -> [w1191]
        tunnel: [w1191] -> w905
        tunnel: w904 -> [w1190]
        tunnel: [w1190] -> w903
        tunnel: w902 -> [w1189]
        tunnel: [w1189] -> w901
        tunnel: w900 -> [w1188]
        tunnel: [w1188] -> w899
        tunnel: w898 -> [w1187]
        tunnel: [w1187] -> w897
        tunnel: w907 -> [w1196]
        tunnel: [w1195] -> w933
        tunnel: w905 -> [w1205]
        tunnel: [w1206] -> w932
        tunnel: w903 -> [w1208]
        tunnel: [w1208] -> w930
        tunnel: w901 -> [w1207]
        tunnel: [w1207] -> w928
        tunnel: [w1200] -> w926
        tunnel: w899 -> [w1199]
        tunnel: [w1198] -> w924
        tunnel: w897 -> [w1201]
        tunnel: w933 -> [w1215]
        tunnel: w932 -> [w1213]
        tunnel: [w1212] -> w931
        tunnel: w930 -> [w1219]
        tunnel: [w1219] -> w929
        tunnel: w928 -> [w1218]
        tunnel: [w1218] -> w927
        tunnel: w926 -> [w1217]
        tunnel: [w1217] -> w925
        tunnel: w924 -> [w1216]
        tunnel: [w1216] -> w923
        tunnel: [w1214] -> w888
        tunnel: [w1230] -> w896
        tunnel: w931 -> [w1227]
        tunnel: w929 -> [w1233]
        tunnel: [w1233] -> w892
        tunnel: w927 -> [w1225]
        tunnel: w925 -> [w1224]
        tunnel: w923 -> [w1222]
        tunnel: w888 -> [w1231]
        tunnel: [w1226] -> w887
        tunnel: [w1225] -> w886
        tunnel: [w1223] -> w885
        tunnel: [w1221] -> w884
        tunnel: w896 -> [w1240]
        tunnel: [w1240] -> w895
        tunnel: [w1239] -> w894
        tunnel: [w1238] -> w893
        tunnel: w892 -> [w1237]
        tunnel: [w1237] -> w891
        tunnel: [w1236] -> w890
        tunnel: [w1235] -> w889
        tunnel: w887 -> [w1239]
        tunnel: w886 -> [w1238]
        tunnel: w885 -> [w1236]
        tunnel: w884 -> [w1235]
        tunnel: w895 -> [w1247]
        tunnel: w894 -> [w1246]
        tunnel: w893 -> [w1244]
        tunnel: w891 -> [w1245]
        tunnel: [w1245] -> w998
        tunnel: [w1244] -> w997
        tunnel: w890 -> [w1243]
        tunnel: w889 -> [w1242]
        tunnel: w998 -> [w1253]
        tunnel: w997 -> [w1251]
        frame #0 {
          n241 = call <vilib>:"WPI_GyroRefNum Registry Get.vi"("refnum name"="AD Gyro") -> ("GyroDevRef"=w1004:T14)  [unwired: 9 in, 1 out]
          n242 = call <vilib>:"WPI_GyroReset.vi"("GyroDevRef"=w1004) -> ()  [unwired: 9 in, 2 out]
          n243 = Wait (ms)(milliseconds to wait=u32 5) -> ()  [unwired: 1 out]
        }
        frame #1 {
          # "Set to shot location"
          n244 = while {
            stop <- TRUE stop-if-true
            n245 = call "Set Shooter Config.vi"("POV Joystick Input"=270) -> ()  [unwired: 3 in]
          }
          n246 = Wait (ms)(milliseconds to wait=u32 5) -> ()  [unwired: 1 out]
        }
        frame #2 {
          # "Intake Pivot out"
          n247 = call <vilib>:"WPI_SolenoidRefNum Registry Get.vi"("refnum name"="Intake Pivot") -> ("error out"=w1018:errorcluster, "SolenoidDevRef"=w1017:T12)  [unwired: 9 in]
          n248 = call-poly <vilib>:"WPI_SolenoidSet.vi"("error in (no error)"=w1018, "Value"=WPI_SolenoidValue."Reverse", "SolenoidDevRef"=w1017) -> ()  [unwired: 7 in, 2 out]
        }
        frame #3 {
          w1020 = 0.7 ("Output")
          n249 = call <vilib>:"WPI_MotorControlRefNum Registry Get.vi"("refnum name"="Intake") -> ("MotorControlDevRef"=w1023:T5)  [unwired: 9 in, 1 out]
          n250 = call <vilib>:"WPI_MotorControlRefNum Registry Get.vi"("refnum name"="Singulator") -> ("MotorControlDevRef"=w1024:T5)  [unwired: 9 in, 1 out]
          n251 = Wait (ms)(milliseconds to wait=u32 10) -> ()  [unwired: 1 out]
          n252 = call <vilib>:"WPI_MotorControlSetOutput.vi"("Output"=w1020, "MotorControlDevRef"=w1024) -> ("MotorControlDevRef"=w1022:T5)  [unwired: 7 in, 2 out]
          n253 = call <vilib>:"WPI_MotorControlSetOutput.vi"("Output"=w1020, "MotorControlDevRef"=w1023) -> ("MotorControlDevRef"=w1021:T5)  [unwired: 7 in, 2 out]
        }
        frame #4 {
          # "Drive away from Hub"
          n254 = Wait (ms)(milliseconds to wait=u32 700) -> ()  [unwired: 1 out]
          n255 = call <vilib>:"WPI_RobotDriveRefNum Registry Get.vi"("refnum name"="6MRobotDrive") -> ("error out"=w1038:errorcluster, "RobotDriveDevRef"=w1037:T4)  [unwired: 1 in, 8 out]
          n256 = call <vilib>:"WPI_RobotDriveArcadeDrive_Standard(NoSaturation).vi"("Y axis value"=0.0, "X axis value"=-0.7, "RobotDriveDevRef"=w1037) -> ()  [unwired: 1 in, 8 out]
          n257 = call <vilib>:"WPI_RobotDriveSafetyConfig.vi"("error in (no error)"=w1038, "mode"=WPI_SafetyOutputConfigMenu."Disable", "RobotDriveDevRef"=w1037) -> ("error out"=w1034:errorcluster, "RobotDriveDevRef"=w1035:T4)  [unwired: 7 in]
        }
        frame #5 {
          # "Drive to Fender and intake"
          n258 = Wait (ms)(milliseconds to wait=u32 550) -> ()  [unwired: 1 out]
          n259 = call <vilib>:"WPI_RobotDriveArcadeDrive_Standard(NoSaturation).vi"("Y axis value"=0.0, "X axis value"=0.7, "RobotDriveDevRef"=w1047) -> ()  [unwired: 1 in, 8 out]
        }
        frame #6 {
          w1054 = 0.0 ("Output")
          # "Drive to fender intake off"
          n260 = Wait (ms)(milliseconds to wait=u32 50) -> ()  [unwired: 1 out]
          n261 = call <vilib>:"WPI_MotorControlSetOutput.vi"("Output"=w1054, "MotorControlDevRef"=w1055) -> ("MotorControlDevRef"=w1052:T5)  [unwired: 7 in, 2 out]
          n262 = call <vilib>:"WPI_MotorControlSetOutput.vi"("Output"=w1054, "MotorControlDevRef"=w1056) -> ("MotorControlDevRef"=w1051:T5)  [unwired: 7 in, 2 out]
        }
        frame #7 {
          n263 = call <vilib>:"WPI_RobotDriveArcadeDrive_Standard(NoSaturation).vi"("error in (no error)"=w1063, "Y axis value"=0.0, "X axis value"=0.0, "RobotDriveDevRef"=w1064) -> ()  [unwired: 8 out]
        }
        frame #8 {
          # "Turn on Shooter"
          n264 = global read "Global Shooter Speed.vi" "Shooter Speed Target"() -> (w1078:dbl)
          n265 = Wait (ms)(milliseconds to wait=u32 500) -> ()  [unwired: 1 out]
          n266 = global read "Global Shooter Speed.vi" "Accelerator Speed Target"() -> (w1076:dbl)
          n267 = call <vilib>:"Spark MAX Set Output Advanced.vi"("Control Mode"=Spark_MAX_Control_Type."Velocity", "Setpoint"=w1078, "MotorControlDevRef"=w1073) -> ("MotorControlDevRef"=w1072:T5)  [unwired: 7 in, 1 out]
          n268 = call <vilib>:"Spark MAX Set Output Advanced.vi"("Control Mode"=Spark_MAX_Control_Type."Velocity", "Setpoint"=w1076, "MotorControlDevRef"=w1075) -> ("MotorControlDevRef"=w1074:T5)  [unwired: 7 in, 1 out]
        }
        frame #9 {
        }
        frame #10 {
          # "Feed"
          n269 = Wait (ms)(milliseconds to wait=u32 2000) -> ()  [unwired: 1 out]
          n270 = call "Feed to Shooter.vi"("Feed Input"=0.3) -> ()  [unwired: 11 in]
        }
        frame #11 {
          n271 = call "Feed to Shooter.vi"("Feed Input"=0.0) -> ()  [unwired: 11 in]
          n272 = Wait (ms)(milliseconds to wait=u32 500) -> ()  [unwired: 1 out]
        }
        frame #12 {
          # "Turn to Angle"
          n273 = while {
            shift-right: [w1119] -> w1112
            shift-left: w1115 -> [w1119]
            shift-right: [w1118] -> w1113
            shift-left: w1114 -> [w1118]
            stop <- w1116 stop-if-true
            n274 = call "Turn to Angle.vi"("Target Angle"=-70.0) -> ("Angle Reached?"=w1116:bool)  [unwired: 10 in]
          }
          n275 = call <vilib>:"WPI_MotorControlSetOutput.vi"("Output"=0.0, "MotorControlDevRef"=w1107) -> ("MotorControlDevRef"=w1106:T5)  [unwired: 7 in, 2 out]
          n276 = call <vilib>:"WPI_MotorControlSetOutput.vi"("Output"=0.0, "MotorControlDevRef"=w1110) -> ("MotorControlDevRef"=w1109:T5)  [unwired: 7 in, 2 out]
        }
        frame #13 {
          w1120 = 0.7 ("Output")
          # "Drive and Pickup"
          n277 = Wait (ms)(milliseconds to wait=u32 1500) -> ()  [unwired: 1 out]
          n278 = call <vilib>:"WPI_RobotDriveArcadeDrive_Standard(NoSaturation).vi"("error in (no error)"=w1128, "Y axis value"=0.0, "X axis value"=-0.7, "RobotDriveDevRef"=w1132) -> ("error out"=w1127:errorcluster, "RobotDriveDevRef"=w1131:T4)  [unwired: 6 out]
          n279 = call <vilib>:"WPI_MotorControlSetOutput.vi"("Output"=w1120, "MotorControlDevRef"=w1123) -> ("MotorControlDevRef"=w1124:T5)  [unwired: 7 in, 2 out]
          n280 = call <vilib>:"WPI_MotorControlSetOutput.vi"("Output"=w1120, "MotorControlDevRef"=w1122) -> ("MotorControlDevRef"=w1121:T5)  [unwired: 7 in, 2 out]
        }
        frame #14 {
          # "Stop Driving"
          n281 = call-poly <vilib>:"WPI_RobotDriveArcadeDrive.vi"("error in (no error)"=w1138, "Y axis value"=0.0, "X axis value"=0.0, "RobotDriveDevRef"=w1142) -> ("error out"=w1137:errorcluster, "RobotDriveDevRef"=w1141:T4)  [unwired: 5 in, 1 out]
          n282 = Wait (ms)(milliseconds to wait=u32 1000) -> ()  [unwired: 1 out]
        }
        frame #15 {
          n283 = while {
            stop <- w1151 stop-if-true
            n284 = call "Turn to Angle.vi"("Target Angle"=-39.0) -> ("Angle Reached?"=w1151:bool)  [unwired: 10 in]
          }
        }
        frame #16 {
          w1153 = 0.0 ("Output")
          # "Set Shooter"
          n285 = while {
            stop <- TRUE stop-if-true
            n286 = call "Set Shooter Config.vi"("POV Joystick Input"=90) -> ()  [unwired: 3 in]
          }
          n287 = call <vilib>:"WPI_MotorControlSetOutput.vi"("Output"=w1153, "MotorControlDevRef"=w1155) -> ("MotorControlDevRef"=w1157:T5)  [unwired: 7 in, 2 out]
          n288 = call <vilib>:"WPI_MotorControlSetOutput.vi"("Output"=w1153, "MotorControlDevRef"=w1154) -> ("MotorControlDevRef"=w1156:T5)  [unwired: 7 in, 2 out]
          n289 = Wait (ms)(milliseconds to wait=u32 50) -> ()  [unwired: 1 out]
        }
        frame #17 {
          # "Turn on Shooter"
          n290 = global read "Global Shooter Speed.vi" "Shooter Speed Target"() -> (w1172:dbl)
          n291 = global read "Global Shooter Speed.vi" "Accelerator Speed Target"() -> (w1170:dbl)
          n292 = Wait (ms)(milliseconds to wait=u32 1000) -> ()  [unwired: 1 out]
          n293 = call <vilib>:"Spark MAX Set Output Advanced.vi"("Control Mode"=Spark_MAX_Control_Type."Velocity", "Setpoint"=w1172, "MotorControlDevRef"=w1169) -> ("MotorControlDevRef"=w1168:T5)  [unwired: 7 in, 1 out]
          n294 = call <vilib>:"Spark MAX Set Output Advanced.vi"("Control Mode"=Spark_MAX_Control_Type."Velocity", "Setpoint"=w1170, "MotorControlDevRef"=w1167) -> ("MotorControlDevRef"=w1166:T5)  [unwired: 7 in, 1 out]
        }
        frame #18 {
          # "Shoot #3"
          n295 = Wait (ms)(milliseconds to wait=u32 2000) -> ()  [unwired: 1 out]
          n296 = call "Feed to Shooter.vi"("Feed Input"=0.3) -> ()  [unwired: 11 in]
        }
        frame #19 {
          n297 = while {
            stop <- w1193 stop-if-true
            n298 = call "Turn to Angle.vi"("Target Angle"=-69.0) -> ("Angle Reached?"=w1193:bool)  [unwired: 10 in]
          }
          n299 = call "Feed to Shooter.vi"("Feed Input"=0.0) -> ()  [unwired: 11 in]
        }
        frame #20 {
          w1197 = 0.7 ("Output")
          # "Pickup?"
          # "Drive to Terminal"
          n300 = call <vilib>:"WPI_RobotDriveArcadeDrive_Standard(NoSaturation).vi"("error in (no error)"=w1205, "Y axis value"=0.0, "X axis value"=-0.7, "RobotDriveDevRef"=w1196) -> ("error out"=w1206:errorcluster, "RobotDriveDevRef"=w1195:T4)  [unwired: 6 out]
          n301 = call <vilib>:"WPI_MotorControlSetOutput.vi"("Output"=w1197, "MotorControlDevRef"=w1201) -> ("MotorControlDevRef"=w1200:T5)  [unwired: 7 in, 2 out]
          n302 = call <vilib>:"WPI_MotorControlSetOutput.vi"("Output"=w1197, "MotorControlDevRef"=w1199) -> ("MotorControlDevRef"=w1198:T5)  [unwired: 7 in, 2 out]
          n303 = Wait (ms)(milliseconds to wait=u32 2850) -> ()  [unwired: 1 out]
        }
        frame #21 {
          # "Drive to Hub?"
          n304 = call <vilib>:"WPI_RobotDriveArcadeDrive_Standard(NoSaturation).vi"("error in (no error)"=w1213, "Y axis value"=-0.2, "X axis value"=0.7, "RobotDriveDevRef"=w1215) -> ("error out"=w1212:errorcluster, "RobotDriveDevRef"=w1214:T4)  [unwired: 6 out]
          n305 = Wait (ms)(milliseconds to wait=u32 2000) -> ()  [unwired: 1 out]
        }
        frame #22 {
          w1220 = 0.0 ("Output")
          # "Stop"
          n306 = call <vilib>:"WPI_RobotDriveArcadeDrive_Standard(NoSaturation).vi"("error in (no error)"=w1227, "Y axis value"=0.0, "X axis value"=0.0, "RobotDriveDevRef"=w1231) -> ("error out"=w1226:errorcluster, "RobotDriveDevRef"=w1230:T4)  [unwired: 6 out]
          n307 = call <vilib>:"WPI_MotorControlSetOutput.vi"("Output"=w1220, "MotorControlDevRef"=w1224) -> ("MotorControlDevRef"=w1223:T5)  [unwired: 7 in, 2 out]
          n308 = call <vilib>:"WPI_MotorControlSetOutput.vi"("Output"=w1220, "MotorControlDevRef"=w1222) -> ("MotorControlDevRef"=w1221:T5)  [unwired: 7 in, 2 out]
          n309 = Wait (ms)(milliseconds to wait=u32 1000) -> ()  [unwired: 1 out]
        }
        frame #23 {
          # "Shoot"
          n310 = call "Feed to Shooter.vi"("Feed Input"=0.3) -> ()  [unwired: 11 in]
        }
        frame #24 {
          w1241 = 0.0 ("Output")
          # "Turn Off"
          n311 = call <vilib>:"WPI_MotorControlSetOutput.vi"("Output"=w1241, "MotorControlDevRef"=w1243) -> ()  [unwired: 7 in, 3 out]
          n312 = call <vilib>:"WPI_MotorControlSetOutput.vi"("Output"=w1241, "MotorControlDevRef"=w1242) -> ()  [unwired: 7 in, 3 out]
          n313 = call <vilib>:"WPI_RobotDriveArcadeDrive_Standard(NoSaturation).vi"("error in (no error)"=w1246, "Y axis value"=0.0, "X axis value"=0.0, "RobotDriveDevRef"=w1247) -> ()  [unwired: 8 out]
          n314 = Wait (ms)(milliseconds to wait=u32 1000) -> ()  [unwired: 1 out]
        }
        frame #25 {
          n315 = call <vilib>:"WPI_MotorControlSetOutput.vi"("Output"=0.0, "MotorControlDevRef"=w1251) -> ()  [unwired: 7 in, 3 out]
          n316 = call <vilib>:"WPI_MotorControlSetOutput.vi"("Output"=0.0, "MotorControlDevRef"=w1253) -> ()  [unwired: 7 in, 3 out]
        }
      }
    }
    frame "Three" {
      n317 = flat-sequence {
        tunnel: w1361 -> [w1368]
        tunnel: w1363 -> [w1369]
        tunnel: [w1369] -> w1360
        tunnel: [w1368] -> w1359
        tunnel: [w1371] -> w1364
        tunnel: [w1370] -> w1362
        tunnel: w1360 -> [w1371]
        tunnel: w1359 -> [w1370]
        tunnel: w1364 -> [w1376]
        tunnel: w1362 -> [w1375]
        tunnel: [w1376] -> w1354
        tunnel: [w1375] -> w1351
        tunnel: [w1390] -> w1355
        tunnel: w1354 -> [w1390]
        tunnel: [w1389] -> w1352
        tunnel: w1351 -> [w1389]
        tunnel: [w1384] -> w1349
        tunnel: [w1383] -> w1347
        tunnel: [w1397] -> w1358
        tunnel: [w1396] -> w1357
        tunnel: [w1394] -> w1356
        tunnel: w1355 -> [w1394]
        tunnel: [w1393] -> w1353
        tunnel: w1352 -> [w1393]
        tunnel: [w1392] -> w1350
        tunnel: w1349 -> [w1392]
        tunnel: [w1391] -> w1348
        tunnel: w1347 -> [w1391]
        tunnel: w1358 -> [w1409]
        tunnel: [w1409] -> w1334
        tunnel: w1357 -> [w1412]
        tunnel: [w1412] -> w1332
        tunnel: [w1406] -> w1330
        tunnel: [w1407] -> w1328
        tunnel: w1356 -> [w1407]
        tunnel: w1353 -> [w1406]
        tunnel: w1350 -> [w1404]
        tunnel: w1348 -> [w1405]
        tunnel: [w1405] -> w1326
        tunnel: [w1404] -> w1325
        tunnel: w1334 -> [w1422]
        tunnel: [w1422] -> w1333
        tunnel: w1332 -> [w1421]
        tunnel: [w1421] -> w1331
        tunnel: w1330 -> [w1420]
        tunnel: [w1420] -> w1329
        tunnel: w1328 -> [w1419]
        tunnel: [w1419] -> w1327
        tunnel: w1326 -> [w1418]
        tunnel: w1325 -> [w1417]
        tunnel: [w1414] -> w1309
        tunnel: [w1413] -> w1302
        tunnel: w1333 -> [w1426]
        tunnel: [w1426] -> w1338
        tunnel: w1331 -> [w1425]
        tunnel: [w1425] -> w1337
        tunnel: w1329 -> [w1430]
        tunnel: [w1430] -> w1336
        tunnel: w1327 -> [w1429]
        tunnel: [w1429] -> w1335
        tunnel: [w1424] -> w1310
        tunnel: w1309 -> [w1424]
        tunnel: [w1423] -> w1303
        tunnel: w1302 -> [w1423]
        tunnel: w1338 -> [w1443]
        tunnel: [w1443] -> w1346
        tunnel: w1337 -> [w1442]
        tunnel: [w1442] -> w1344
        tunnel: [w1434] -> w1342
        tunnel: w1336 -> [w1437]
        tunnel: [w1436] -> w1340
        tunnel: w1335 -> [w1435]
        tunnel: [w1433] -> w1311
        tunnel: w1310 -> [w1433]
        tunnel: [w1432] -> w1304
        tunnel: w1303 -> [w1432]
        tunnel: w1346 -> [w1449]
        tunnel: [w1449] -> w1345
        tunnel: w1344 -> [w1448]
        tunnel: [w1448] -> w1343
        tunnel: w1342 -> [w1447]
        tunnel: [w1447] -> w1341
        tunnel: w1340 -> [w1446]
        tunnel: [w1446] -> w1339
        tunnel: [w1445] -> w1312
        tunnel: w1311 -> [w1445]
        tunnel: [w1444] -> w1305
        tunnel: w1304 -> [w1444]
        tunnel: w1345 -> [w1457]
        tunnel: [w1457] -> w1324
        tunnel: w1343 -> [w1456]
        tunnel: [w1456] -> w1322
        tunnel: w1341 -> [w1455]
        tunnel: [w1455] -> w1320
        tunnel: w1339 -> [w1454]
        tunnel: [w1454] -> w1318
        tunnel: [w1451] -> w1313
        tunnel: w1312 -> [w1451]
        tunnel: [w1450] -> w1306
        tunnel: w1305 -> [w1450]
        tunnel: w1324 -> [w1465]
        tunnel: [w1465] -> w1323
        tunnel: w1322 -> [w1464]
        tunnel: [w1464] -> w1321
        tunnel: w1320 -> [w1463]
        tunnel: [w1463] -> w1319
        tunnel: w1318 -> [w1462]
        tunnel: [w1462] -> w1317
        tunnel: [w1460] -> w1314
        tunnel: w1313 -> [w1460]
        tunnel: [w1459] -> w1307
        tunnel: w1306 -> [w1459]
        tunnel: w1323 -> [w1477]
        tunnel: w1321 -> [w1476]
        tunnel: [w1475] -> w1316
        tunnel: w1319 -> [w1469]
        tunnel: w1317 -> [w1472]
        tunnel: [w1474] -> w1315
        tunnel: w1314 -> [w1466]
        tunnel: [w1473] -> w1308
        tunnel: w1307 -> [w1473]
        tunnel: [w1471] -> w1285
        tunnel: [w1468] -> w1284
        tunnel: [w1466] -> w1276
        tunnel: [w1493] -> w1301
        tunnel: w1316 -> [w1490]
        tunnel: [w1489] -> w1300
        tunnel: [w1495] -> w1299
        tunnel: w1315 -> [w1494]
        tunnel: w1308 -> [w1484]
        tunnel: [w1487] -> w1298
        tunnel: w1285 -> [w1495]
        tunnel: w1284 -> [w1487]
        tunnel: [w1486] -> w1277
        tunnel: w1276 -> [w1485]
        tunnel: [w1483] -> w1275
        tunnel: w1301 -> [w1504]
        tunnel: [w1503] -> w1291
        tunnel: w1300 -> [w1500]
        tunnel: [w1499] -> w1290
        tunnel: w1299 -> [w1506]
        tunnel: [w1506] -> w1289
        tunnel: w1298 -> [w1505]
        tunnel: [w1505] -> w1288
        tunnel: [w1496] -> w1287
        tunnel: [w1497] -> w1286
        tunnel: w1277 -> [w1497]
        tunnel: w1275 -> [w1496]
        tunnel: w1291 -> [w1512]
        tunnel: [w1512] -> w1274
        tunnel: w1290 -> [w1511]
        tunnel: [w1511] -> w1273
        tunnel: w1289 -> [w1510]
        tunnel: [w1510] -> w1271
        tunnel: w1288 -> [w1509]
        tunnel: [w1509] -> w1269
        tunnel: w1287 -> [w1508]
        tunnel: [w1508] -> w1267
        tunnel: w1286 -> [w1507]
        tunnel: [w1507] -> w1265
        tunnel: w1274 -> [w1521]
        tunnel: w1273 -> [w1519]
        tunnel: [w1518] -> w1272
        tunnel: w1271 -> [w1525]
        tunnel: [w1525] -> w1270
        tunnel: w1269 -> [w1524]
        tunnel: [w1524] -> w1268
        tunnel: w1267 -> [w1523]
        tunnel: [w1523] -> w1266
        tunnel: w1265 -> [w1522]
        tunnel: [w1522] -> w1264
        tunnel: [w1520] -> w1263
        tunnel: [w1528] -> w1283
        tunnel: w1272 -> [w1526]
        tunnel: [w1527] -> w1282
        tunnel: w1270 -> [w1539]
        tunnel: [w1539] -> w1281
        tunnel: w1268 -> [w1538]
        tunnel: [w1538] -> w1280
        tunnel: w1266 -> [w1533]
        tunnel: [w1535] -> w1279
        tunnel: w1264 -> [w1534]
        tunnel: [w1536] -> w1278
        tunnel: w1263 -> [w1529]
        tunnel: w1283 -> [w1552]
        tunnel: [w1552] -> w1297
        tunnel: w1282 -> [w1551]
        tunnel: [w1551] -> w1296
        tunnel: w1281 -> [w1542]
        tunnel: [w1541] -> w1295
        tunnel: w1280 -> [w1544]
        tunnel: [w1543] -> w1294
        tunnel: w1279 -> [w1550]
        tunnel: [w1550] -> w1293
        tunnel: w1278 -> [w1549]
        tunnel: [w1549] -> w1292
        tunnel: w1297 -> [w1556]
        tunnel: w1296 -> [w1555]
        tunnel: w1295 -> [w1560]
        tunnel: [w1560] -> w1262
        tunnel: w1294 -> [w1559]
        tunnel: [w1559] -> w1261
        tunnel: w1293 -> [w1553]
        tunnel: w1292 -> [w1554]
        tunnel: [w1556] -> w1260
        tunnel: [w1555] -> w1259
        tunnel: [w1554] -> w1258
        tunnel: [w1553] -> w1257
        tunnel: w1262 -> [w1570]
        tunnel: [w1570] -> w1255
        tunnel: w1261 -> [w1566]
        tunnel: [w1566] -> w1256
        tunnel: w1260 -> [w1564]
        tunnel: w1259 -> [w1563]
        tunnel: w1258 -> [w1562]
        tunnel: w1257 -> [w1561]
        tunnel: w1255 -> [w1573]
        tunnel: w1256 -> [w1571]
        frame #0 {
          n318 = call <vilib>:"WPI_GyroRefNum Registry Get.vi"("refnum name"="AD Gyro") -> ("GyroDevRef"=w1366:T14)  [unwired: 9 in, 1 out]
          n319 = call <vilib>:"WPI_GyroReset.vi"("GyroDevRef"=w1366) -> ()  [unwired: 9 in, 2 out]
          n320 = Wait (ms)(milliseconds to wait=u32 5) -> ()  [unwired: 1 out]
        }
        frame #1 {
          # "Set to shot location"
          n321 = while {
            stop <- TRUE stop-if-true
            n322 = call "Set Shooter Config.vi"("POV Joystick Input"=270) -> ()  [unwired: 3 in]
          }
          n323 = Wait (ms)(milliseconds to wait=u32 5) -> ()  [unwired: 1 out]
        }
        frame #2 {
          # "Intake Pivot out"
          n324 = call <vilib>:"WPI_SolenoidRefNum Registry Get.vi"("refnum name"="Intake Pivot") -> ("error out"=w1380:errorcluster, "SolenoidDevRef"=w1379:T12)  [unwired: 9 in]
          n325 = call-poly <vilib>:"WPI_SolenoidSet.vi"("error in (no error)"=w1380, "Value"=WPI_SolenoidValue."Reverse", "SolenoidDevRef"=w1379) -> ()  [unwired: 7 in, 2 out]
        }
        frame #3 {
          w1382 = 0.7 ("Output")
          n326 = call <vilib>:"WPI_MotorControlRefNum Registry Get.vi"("refnum name"="Intake") -> ("MotorControlDevRef"=w1385:T5)  [unwired: 9 in, 1 out]
          n327 = call <vilib>:"WPI_MotorControlRefNum Registry Get.vi"("refnum name"="Singulator") -> ("MotorControlDevRef"=w1386:T5)  [unwired: 9 in, 1 out]
          n328 = Wait (ms)(milliseconds to wait=u32 10) -> ()  [unwired: 1 out]
          n329 = call <vilib>:"WPI_MotorControlSetOutput.vi"("Output"=w1382, "MotorControlDevRef"=w1386) -> ("MotorControlDevRef"=w1384:T5)  [unwired: 7 in, 2 out]
          n330 = call <vilib>:"WPI_MotorControlSetOutput.vi"("Output"=w1382, "MotorControlDevRef"=w1385) -> ("MotorControlDevRef"=w1383:T5)  [unwired: 7 in, 2 out]
        }
        frame #4 {
          # "Drive away from Hub"
          n331 = Wait (ms)(milliseconds to wait=u32 700) -> ()  [unwired: 1 out]
          n332 = call <vilib>:"WPI_RobotDriveRefNum Registry Get.vi"("refnum name"="6MRobotDrive") -> ("error out"=w1400:errorcluster, "RobotDriveDevRef"=w1399:T4)  [unwired: 1 in, 8 out]
          n333 = call <vilib>:"WPI_RobotDriveArcadeDrive_Standard(NoSaturation).vi"("Y axis value"=0.0, "X axis value"=-0.7, "RobotDriveDevRef"=w1399) -> ()  [unwired: 1 in, 8 out]
          n334 = call <vilib>:"WPI_RobotDriveSafetyConfig.vi"("error in (no error)"=w1400, "mode"=WPI_SafetyOutputConfigMenu."Disable", "RobotDriveDevRef"=w1399) -> ("error out"=w1396:errorcluster, "RobotDriveDevRef"=w1397:T4)  [unwired: 7 in]
        }
        frame #5 {
          # "Drive to Fender and intake"
          n335 = Wait (ms)(milliseconds to wait=u32 550) -> ()  [unwired: 1 out]
          n336 = call <vilib>:"WPI_RobotDriveArcadeDrive_Standard(NoSaturation).vi"("Y axis value"=0.0, "X axis value"=0.7, "RobotDriveDevRef"=w1409) -> ()  [unwired: 1 in, 8 out]
        }
        frame #6 {
          w1416 = 0.0 ("Output")
          # "Drive to fender intake off"
          n337 = Wait (ms)(milliseconds to wait=u32 50) -> ()  [unwired: 1 out]
          n338 = call <vilib>:"WPI_MotorControlSetOutput.vi"("Output"=w1416, "MotorControlDevRef"=w1417) -> ("MotorControlDevRef"=w1414:T5)  [unwired: 7 in, 2 out]
          n339 = call <vilib>:"WPI_MotorControlSetOutput.vi"("Output"=w1416, "MotorControlDevRef"=w1418) -> ("MotorControlDevRef"=w1413:T5)  [unwired: 7 in, 2 out]
        }
        frame #7 {
          n340 = call <vilib>:"WPI_RobotDriveArcadeDrive_Standard(NoSaturation).vi"("error in (no error)"=w1425, "Y axis value"=0.0, "X axis value"=0.0, "RobotDriveDevRef"=w1426) -> ()  [unwired: 8 out]
        }
        frame #8 {
          # "Turn on Shooter"
          n341 = global read "Global Shooter Speed.vi" "Shooter Speed Target"() -> (w1440:dbl)
          n342 = Wait (ms)(milliseconds to wait=u32 500) -> ()  [unwired: 1 out]
          n343 = global read "Global Shooter Speed.vi" "Accelerator Speed Target"() -> (w1438:dbl)
          n344 = call <vilib>:"Spark MAX Set Output Advanced.vi"("Control Mode"=Spark_MAX_Control_Type."Velocity", "Setpoint"=w1440, "MotorControlDevRef"=w1435) -> ("MotorControlDevRef"=w1434:T5)  [unwired: 7 in, 1 out]
          n345 = call <vilib>:"Spark MAX Set Output Advanced.vi"("Control Mode"=Spark_MAX_Control_Type."Velocity", "Setpoint"=w1438, "MotorControlDevRef"=w1437) -> ("MotorControlDevRef"=w1436:T5)  [unwired: 7 in, 1 out]
        }
        frame #9 {
        }
        frame #10 {
          # "Feed"
          n346 = Wait (ms)(milliseconds to wait=u32 2000) -> ()  [unwired: 1 out]
          n347 = call "Feed to Shooter.vi"("Feed Input"=0.3) -> ()  [unwired: 11 in]
        }
        frame #11 {
          n348 = call "Feed to Shooter.vi"("Feed Input"=0.0) -> ()  [unwired: 11 in]
          n349 = Wait (ms)(milliseconds to wait=u32 500) -> ()  [unwired: 1 out]
        }
        frame #12 {
          # "Turn to Angle"
          n350 = while {
            shift-right: [w1481] -> w1474
            shift-left: w1477 -> [w1481]
            shift-right: [w1480] -> w1475
            shift-left: w1476 -> [w1480]
            stop <- w1478 stop-if-true
            n351 = call "Turn to Angle.vi"("Target Angle"=-65.0) -> ("Angle Reached?"=w1478:bool)  [unwired: 10 in]
          }
          n352 = call <vilib>:"WPI_MotorControlSetOutput.vi"("Output"=0.0, "MotorControlDevRef"=w1469) -> ("MotorControlDevRef"=w1468:T5)  [unwired: 7 in, 2 out]
          n353 = call <vilib>:"WPI_MotorControlSetOutput.vi"("Output"=0.0, "MotorControlDevRef"=w1472) -> ("MotorControlDevRef"=w1471:T5)  [unwired: 7 in, 2 out]
        }
        frame #13 {
          w1482 = 0.7 ("Output")
          # "Drive and Pickup"
          n354 = Wait (ms)(milliseconds to wait=u32 1500) -> ()  [unwired: 1 out]
          n355 = call <vilib>:"WPI_RobotDriveArcadeDrive_Standard(NoSaturation).vi"("error in (no error)"=w1490, "Y axis value"=0.0, "X axis value"=-0.7, "RobotDriveDevRef"=w1494) -> ("error out"=w1489:errorcluster, "RobotDriveDevRef"=w1493:T4)  [unwired: 6 out]
          n356 = call <vilib>:"WPI_MotorControlSetOutput.vi"("Output"=w1482, "MotorControlDevRef"=w1485) -> ("MotorControlDevRef"=w1486:T5)  [unwired: 7 in, 2 out]
          n357 = call <vilib>:"WPI_MotorControlSetOutput.vi"("Output"=w1482, "MotorControlDevRef"=w1484) -> ("MotorControlDevRef"=w1483:T5)  [unwired: 7 in, 2 out]
        }
        frame #14 {
          # "go back"
          n358 = call-poly <vilib>:"WPI_RobotDriveArcadeDrive.vi"("error in (no error)"=w1500, "Y axis value"=0.0, "X axis value"=0.7, "RobotDriveDevRef"=w1504) -> ("error out"=w1499:errorcluster, "RobotDriveDevRef"=w1503:T4)  [unwired: 5 in, 1 out]
          n359 = Wait (ms)(milliseconds to wait=u32 1500) -> ()  [unwired: 1 out]
        }
        frame #15 {
          n360 = while {
            stop <- w1513 stop-if-true
            n361 = call "Turn to Angle.vi"("Target Angle"=0.0) -> ("Angle Reached?"=w1513:bool)  [unwired: 10 in]
          }
        }
        frame #16 {
          n362 = Wait (ms)(milliseconds to wait=u32 50) -> ()  [unwired: 1 out]
          n363 = call-poly <vilib>:"WPI_RobotDriveArcadeDrive.vi"("error in (no error)"=w1519, "Y axis value"=0.0, "X axis value"=0.0, "RobotDriveDevRef"=w1521) -> ("error out"=w1518:errorcluster, "RobotDriveDevRef"=w1520:T4)  [unwired: 5 in, 1 out]
        }
        frame #17 {
          w1532 = 0.0 ("Output")
          n364 = call <vilib>:"WPI_MotorControlSetOutput.vi"("Output"=w1532, "MotorControlDevRef"=w1534) -> ("MotorControlDevRef"=w1536:T5)  [unwired: 7 in, 2 out]
          n365 = call-poly <vilib>:"WPI_RobotDriveArcadeDrive.vi"("error in (no error)"=w1526, "Y axis value"=0.0, "X axis value"=0.0, "RobotDriveDevRef"=w1529) -> ("error out"=w1527:errorcluster, "RobotDriveDevRef"=w1528:T4)  [unwired: 5 in, 1 out]
          n366 = call <vilib>:"WPI_MotorControlSetOutput.vi"("Output"=w1532, "MotorControlDevRef"=w1533) -> ("MotorControlDevRef"=w1535:T5)  [unwired: 7 in, 2 out]
          n367 = Wait (ms)(milliseconds to wait=u32 50) -> ()  [unwired: 1 out]
        }
        frame #18 {
          # "Turn on Shooter"
          n368 = global read "Global Shooter Speed.vi" "Shooter Speed Target"() -> (w1547:dbl)
          n369 = global read "Global Shooter Speed.vi" "Accelerator Speed Target"() -> (w1545:dbl)
          n370 = Wait (ms)(milliseconds to wait=u32 1000) -> ()  [unwired: 1 out]
          n371 = call <vilib>:"Spark MAX Set Output Advanced.vi"("Control Mode"=Spark_MAX_Control_Type."Velocity", "Setpoint"=w1547, "MotorControlDevRef"=w1544) -> ("MotorControlDevRef"=w1543:T5)  [unwired: 7 in, 1 out]
          n372 = call <vilib>:"Spark MAX Set Output Advanced.vi"("Control Mode"=Spark_MAX_Control_Type."Velocity", "Setpoint"=w1545, "MotorControlDevRef"=w1542) -> ("MotorControlDevRef"=w1541:T5)  [unwired: 7 in, 1 out]
        }
        frame #19 {
          # "Shoot #3"
          n373 = Wait (ms)(milliseconds to wait=u32 2000) -> ()  [unwired: 1 out]
          n374 = call "Feed to Shooter.vi"("Feed Input"=0.3) -> ()  [unwired: 11 in]
        }
        frame #20 {
          w1565 = 0.0 ("Output")
          # "Stop"
          n375 = call <vilib>:"WPI_MotorControlSetOutput.vi"("Output"=w1565, "MotorControlDevRef"=w1562) -> ()  [unwired: 7 in, 3 out]
          n376 = call <vilib>:"WPI_MotorControlSetOutput.vi"("Output"=w1565, "MotorControlDevRef"=w1561) -> ()  [unwired: 7 in, 3 out]
          n377 = Wait (ms)(milliseconds to wait=u32 1000) -> ()  [unwired: 1 out]
          n378 = call <vilib>:"WPI_RobotDriveArcadeDrive_Standard(NoSaturation).vi"("error in (no error)"=w1563, "Y axis value"=0.0, "X axis value"=0.0, "RobotDriveDevRef"=w1564) -> ()  [unwired: 8 out]
        }
        frame #21 {
          n379 = call <vilib>:"WPI_MotorControlSetOutput.vi"("Output"=0.0, "MotorControlDevRef"=w1571) -> ()  [unwired: 7 in, 3 out]
          n380 = call <vilib>:"WPI_MotorControlSetOutput.vi"("Output"=0.0, "MotorControlDevRef"=w1573) -> ()  [unwired: 7 in, 3 out]
        }
      }
    }
    frame "Buddy" {
      n381 = flat-sequence {
        tunnel: w1663 -> [w1668]
        tunnel: w1665 -> [w1669]
        tunnel: [w1669] -> w1660
        tunnel: [w1668] -> w1659
        tunnel: [w1671] -> w1666
        tunnel: [w1670] -> w1664
        tunnel: w1660 -> [w1671]
        tunnel: w1659 -> [w1670]
        tunnel: w1666 -> [w1676]
        tunnel: w1664 -> [w1675]
        tunnel: [w1676] -> w1657
        tunnel: [w1675] -> w1655
        tunnel: [w1690] -> w1658
        tunnel: w1657 -> [w1690]
        tunnel: [w1689] -> w1656
        tunnel: w1655 -> [w1689]
        tunnel: [w1684] -> w1654
        tunnel: [w1683] -> w1653
        tunnel: [w1697] -> w1604
        tunnel: [w1696] -> w1603
        tunnel: [w1694] -> w1601
        tunnel: w1658 -> [w1694]
        tunnel: [w1693] -> w1602
        tunnel: w1656 -> [w1693]
        tunnel: [w1692] -> w1600
        tunnel: w1654 -> [w1692]
        tunnel: [w1691] -> w1599
        tunnel: w1653 -> [w1691]
        tunnel: w1604 -> [w1712]
        tunnel: [w1712] -> w1640
        tunnel: w1603 -> [w1711]
        tunnel: [w1711] -> w1639
        tunnel: w1602 -> [w1710]
        tunnel: [w1710] -> w1638
        tunnel: w1601 -> [w1709]
        tunnel: [w1709] -> w1637
        tunnel: w1599 -> [w1708]
        tunnel: w1600 -> [w1707]
        tunnel: [w1705] -> w1618
        tunnel: [w1704] -> w1611
        tunnel: w1640 -> [w1716]
        tunnel: [w1716] -> w1644
        tunnel: w1639 -> [w1715]
        tunnel: [w1715] -> w1643
        tunnel: w1638 -> [w1720]
        tunnel: [w1720] -> w1642
        tunnel: w1637 -> [w1719]
        tunnel: [w1719] -> w1641
        tunnel: [w1714] -> w1619
        tunnel: w1618 -> [w1714]
        tunnel: [w1713] -> w1612
        tunnel: w1611 -> [w1713]
        tunnel: w1644 -> [w1732]
        tunnel: [w1732] -> w1652
        tunnel: w1643 -> [w1731]
        tunnel: [w1731] -> w1650
        tunnel: [w1723] -> w1648
        tunnel: w1642 -> [w1726]
        tunnel: [w1725] -> w1646
        tunnel: w1641 -> [w1724]
        tunnel: [w1722] -> w1620
        tunnel: w1619 -> [w1722]
        tunnel: [w1721] -> w1613
        tunnel: w1612 -> [w1721]
        tunnel: w1652 -> [w1739]
        tunnel: [w1739] -> w1651
        tunnel: w1650 -> [w1738]
        tunnel: [w1738] -> w1649
        tunnel: w1648 -> [w1737]
        tunnel: [w1737] -> w1647
        tunnel: w1646 -> [w1736]
        tunnel: [w1736] -> w1645
        tunnel: [w1734] -> w1621
        tunnel: w1620 -> [w1734]
        tunnel: [w1733] -> w1614
        tunnel: w1613 -> [w1733]
        tunnel: w1651 -> [w1747]
        tunnel: [w1747] -> w1636
        tunnel: w1649 -> [w1746]
        tunnel: [w1746] -> w1634
        tunnel: w1647 -> [w1745]
        tunnel: [w1745] -> w1632
        tunnel: w1645 -> [w1744]
        tunnel: [w1744] -> w1630
        tunnel: [w1741] -> w1622
        tunnel: w1621 -> [w1741]
        tunnel: [w1740] -> w1615
        tunnel: w1614 -> [w1740]
        tunnel: w1636 -> [w1760]
        tunnel: [w1760] -> w1635
        tunnel: w1634 -> [w1759]
        tunnel: [w1759] -> w1633
        tunnel: w1632 -> [w1753]
        tunnel: [w1752] -> w1631
        tunnel: w1630 -> [w1750]
        tunnel: [w1749] -> w1629
        tunnel: [w1755] -> w1623
        tunnel: w1622 -> [w1755]
        tunnel: [w1754] -> w1616
        tunnel: w1615 -> [w1754]
        tunnel: w1635 -> [w1766]
        tunnel: w1633 -> [w1765]
        tunnel: [w1764] -> w1628
        tunnel: w1631 -> [w1768]
        tunnel: [w1768] -> w1627
        tunnel: w1629 -> [w1767]
        tunnel: [w1767] -> w1626
        tunnel: [w1763] -> w1625
        tunnel: [w1762] -> w1624
        tunnel: w1623 -> [w1762]
        tunnel: [w1761] -> w1617
        tunnel: w1616 -> [w1761]
        tunnel: [w1784] -> w1598
        tunnel: w1628 -> [w1781]
        tunnel: [w1780] -> w1597
        tunnel: w1627 -> [w1777]
        tunnel: w1626 -> [w1786]
        tunnel: [w1786] -> w1596
        tunnel: w1625 -> [w1785]
        tunnel: w1624 -> [w1773]
        tunnel: w1617 -> [w1778]
        tunnel: [w1777] -> w1595
        tunnel: [w1775] -> w1594
        tunnel: [w1774] -> w1593
        tunnel: w1598 -> [w1790]
        tunnel: [w1789] -> w1592
        tunnel: w1597 -> [w1794]
        tunnel: [w1795] -> w1591
        tunnel: w1596 -> [w1797]
        tunnel: [w1797] -> w1590
        tunnel: w1595 -> [w1796]
        tunnel: [w1796] -> w1589
        tunnel: [w1788] -> w1588
        tunnel: [w1787] -> w1587
        tunnel: w1594 -> [w1788]
        tunnel: w1593 -> [w1787]
        tunnel: w1592 -> [w1803]
        tunnel: w1591 -> [w1799]
        tunnel: [w1798] -> w1586
        tunnel: w1590 -> [w1807]
        tunnel: w1589 -> [w1805]
        tunnel: [w1804] -> w1584
        tunnel: w1588 -> [w1813]
        tunnel: [w1813] -> w1582
        tunnel: w1587 -> [w1812]
        tunnel: [w1812] -> w1580
        tunnel: [w1806] -> w1578
        tunnel: [w1802] -> w1576
        tunnel: w1586 -> [w1820]
        tunnel: [w1820] -> w1585
        tunnel: w1584 -> [w1819]
        tunnel: [w1819] -> w1583
        tunnel: w1582 -> [w1818]
        tunnel: [w1818] -> w1581
        tunnel: w1580 -> [w1817]
        tunnel: [w1817] -> w1579
        tunnel: w1578 -> [w1816]
        tunnel: [w1816] -> w1577
        tunnel: w1576 -> [w1815]
        tunnel: [w1815] -> w1575
        tunnel: [w1828] -> w1610
        tunnel: w1585 -> [w1827]
        tunnel: [w1827] -> w1609
        tunnel: [w1826] -> w1608
        tunnel: [w1825] -> w1607
        tunnel: w1583 -> [w1826]
        tunnel: [w1823] -> w1606
        tunnel: [w1822] -> w1605
        tunnel: w1581 -> [w1823]
        tunnel: w1579 -> [w1822]
        tunnel: w1577 -> [w1825]
        tunnel: w1575 -> [w1828]
        tunnel: w1610 -> [w1835]
        tunnel: w1609 -> [w1834]
        tunnel: w1608 -> [w1832]
        tunnel: w1607 -> [w1833]
        tunnel: [w1833] -> w1662
        tunnel: [w1832] -> w1661
        tunnel: w1606 -> [w1831]
        tunnel: w1605 -> [w1830]
        tunnel: w1662 -> [w1841]
        tunnel: w1661 -> [w1839]
        frame #0 {
          n382 = Wait (ms)(milliseconds to wait=u32 10) -> ()  [unwired: 1 out]
        }
        frame #1 {
          # "Set to shot location"
          n383 = while {
            stop <- TRUE stop-if-true
            n384 = call "Set Shooter Config.vi"("POV Joystick Input"=0) -> ()  [unwired: 3 in]
          }
          n385 = Wait (ms)(milliseconds to wait=u32 10) -> ()  [unwired: 1 out]
        }
        frame #2 {
          # "Intake Pivot out"
          n386 = call <vilib>:"WPI_SolenoidRefNum Registry Get.vi"("refnum name"="Intake Pivot") -> ("error out"=w1680:errorcluster, "SolenoidDevRef"=w1679:T12)  [unwired: 9 in]
          n387 = call-poly <vilib>:"WPI_SolenoidSet.vi"("error in (no error)"=w1680, "Value"=WPI_SolenoidValue."Reverse", "SolenoidDevRef"=w1679) -> ()  [unwired: 7 in, 2 out]
        }
        frame #3 {
          w1682 = 0.7 ("Output")
          n388 = call <vilib>:"WPI_MotorControlRefNum Registry Get.vi"("refnum name"="Intake") -> ("MotorControlDevRef"=w1685:T5)  [unwired: 9 in, 1 out]
          n389 = call <vilib>:"WPI_MotorControlRefNum Registry Get.vi"("refnum name"="Singulator") -> ("MotorControlDevRef"=w1686:T5)  [unwired: 9 in, 1 out]
          n390 = Wait (ms)(milliseconds to wait=u32 10) -> ()  [unwired: 1 out]
          n391 = call <vilib>:"WPI_MotorControlSetOutput.vi"("Output"=w1682, "MotorControlDevRef"=w1686) -> ("MotorControlDevRef"=w1684:T5)  [unwired: 7 in, 2 out]
          n392 = call <vilib>:"WPI_MotorControlSetOutput.vi"("Output"=w1682, "MotorControlDevRef"=w1685) -> ("MotorControlDevRef"=w1683:T5)  [unwired: 7 in, 2 out]
        }
        frame #4 {
          # "Drive away from Hub"
          n393 = Wait (ms)(milliseconds to wait=u32 550) -> ()  [unwired: 1 out]
          n394 = call <vilib>:"WPI_RobotDriveRefNum Registry Get.vi"("refnum name"="6MRobotDrive") -> ("error out"=w1700:errorcluster, "RobotDriveDevRef"=w1699:T4)  [unwired: 1 in, 8 out]
          n395 = call <vilib>:"WPI_RobotDriveArcadeDrive_Standard(NoSaturation).vi"("Y axis value"=0.0, "X axis value"=-0.7, "RobotDriveDevRef"=w1699) -> ()  [unwired: 1 in, 8 out]
          n396 = call <vilib>:"WPI_RobotDriveSafetyConfig.vi"("error in (no error)"=w1700, "mode"=WPI_SafetyOutputConfigMenu."Disable", "RobotDriveDevRef"=w1699) -> ("error out"=w1696:errorcluster, "RobotDriveDevRef"=w1697:T4)  [unwired: 7 in]
        }
        frame #5 {
          w1706 = 0.0 ("Output")
          # "Stop Intaking"
          n397 = call <vilib>:"WPI_MotorControlSetOutput.vi"("Output"=w1706, "MotorControlDevRef"=w1707) -> ("MotorControlDevRef"=w1705:T5)  [unwired: 7 in, 2 out]
          n398 = call <vilib>:"WPI_MotorControlSetOutput.vi"("Output"=w1706, "MotorControlDevRef"=w1708) -> ("MotorControlDevRef"=w1704:T5)  [unwired: 7 in, 2 out]
        }
        frame #6 {
          # "Stop Driving"
          n399 = call <vilib>:"WPI_RobotDriveArcadeDrive_Standard(NoSaturation).vi"("error in (no error)"=w1715, "Y axis value"=0.0, "X axis value"=0.0, "RobotDriveDevRef"=w1716) -> ()  [unwired: 8 out]
        }
        frame #7 {
          # "Turn on Shooter"
          n400 = global read "Global Shooter Speed.vi" "Shooter Speed Target"() -> (w1729:dbl)
          n401 = global read "Global Shooter Speed.vi" "Accelerator Speed Target"() -> (w1727:dbl)
          n402 = call <vilib>:"Spark MAX Set Output Advanced.vi"("Control Mode"=Spark_MAX_Control_Type."Velocity", "Setpoint"=w1729, "MotorControlDevRef"=w1724) -> ("MotorControlDevRef"=w1723:T5)  [unwired: 7 in, 1 out]
          n403 = call <vilib>:"Spark MAX Set Output Advanced.vi"("Control Mode"=Spark_MAX_Control_Type."Velocity", "Setpoint"=w1727, "MotorControlDevRef"=w1726) -> ("MotorControlDevRef"=w1725:T5)  [unwired: 7 in, 1 out]
        }
        frame #8 {
          n404 = Wait (ms)(milliseconds to wait=u32 1000) -> ()  [unwired: 1 out]
        }
        frame #9 {
          # "Feed"
          n405 = Wait (ms)(milliseconds to wait=u32 2000) -> ()  [unwired: 1 out]
          n406 = call "Feed to Shooter.vi"("Feed Input"=0.3) -> ()  [unwired: 11 in]
        }
        frame #10 {
          # "Set Gyro, turn off shooter"
          n407 = call <vilib>:"WPI_MotorControlSetOutput.vi"("Output"=0.0, "MotorControlDevRef"=w1753) -> ("MotorControlDevRef"=w1752:T5)  [unwired: 7 in, 2 out]
          n408 = call <vilib>:"WPI_MotorControlSetOutput.vi"("Output"=0.0, "MotorControlDevRef"=w1750) -> ("MotorControlDevRef"=w1749:T5)  [unwired: 7 in, 2 out]
          n409 = call <vilib>:"WPI_GyroRefNum Registry Get.vi"("refnum name"="AD Gyro") -> ("GyroDevRef"=w1758:T14)  [unwired: 9 in, 1 out]
          n410 = call "Feed to Shooter.vi"("Feed Input"=0.0) -> ()  [unwired: 11 in]
          n411 = call <vilib>:"WPI_GyroReset.vi"("GyroDevRef"=w1758) -> ()  [unwired: 9 in, 2 out]
        }
        frame #11 {
          # "Turn to Angle"
          n412 = while {
            shift-right: [w1769] -> w1763
            shift-left: w1766 -> [w1769]
            shift-right: [w1770] -> w1764
            shift-left: w1765 -> [w1770]
            stop <- w1772 stop-if-true
            n413 = call "Turn to Angle.vi"("Target Angle"=85.0) -> ("Angle Reached?"=w1772:bool)  [unwired: 10 in]
          }
        }
        frame #12 {
          w1776 = 0.7 ("Output")
          # "Drive and Pickup"
          n414 = call <vilib>:"WPI_MotorControlSetOutput.vi"("Output"=w1776, "MotorControlDevRef"=w1778) -> ("MotorControlDevRef"=w1774:T5)  [unwired: 7 in, 2 out]
          n415 = Wait (ms)(milliseconds to wait=u32 3800) -> ()  [unwired: 1 out]
          n416 = call <vilib>:"WPI_RobotDriveArcadeDrive_Standard(NoSaturation).vi"("error in (no error)"=w1781, "Y axis value"=0.0, "X axis value"=-0.7, "RobotDriveDevRef"=w1785) -> ("error out"=w1780:errorcluster, "RobotDriveDevRef"=w1784:T4)  [unwired: 6 out]
          n417 = call <vilib>:"WPI_MotorControlSetOutput.vi"("Output"=w1776, "MotorControlDevRef"=w1773) -> ("MotorControlDevRef"=w1775:T5)  [unwired: 7 in, 2 out]
        }
        frame #13 {
          # "Drive Back"
          n418 = call <vilib>:"WPI_RobotDriveArcadeDrive_Standard(NoSaturation).vi"("error in (no error)"=w1794, "Y axis value"=0.28, "X axis value"=0.7, "RobotDriveDevRef"=w1790) -> ("error out"=w1795:errorcluster, "RobotDriveDevRef"=w1789:T4)  [unwired: 6 out]
          n419 = Wait (ms)(milliseconds to wait=u32 1500) -> ()  [unwired: 1 out]
        }
        frame #14 {
          n420 = global read "Global Shooter Speed.vi" "Shooter Speed Target"() -> (w1810:dbl)
          n421 = global read "Global Shooter Speed.vi" "Accelerator Speed Target"() -> (w1808:dbl)
          n422 = call <vilib>:"WPI_RobotDriveArcadeDrive_Standard(NoSaturation).vi"("error in (no error)"=w1799, "Y axis value"=0.0, "X axis value"=0.0, "RobotDriveDevRef"=w1803) -> ("error out"=w1798:errorcluster, "RobotDriveDevRef"=w1802:T4)  [unwired: 6 out]
          n423 = call <vilib>:"Spark MAX Set Output Advanced.vi"("Control Mode"=Spark_MAX_Control_Type."Velocity", "Setpoint"=w1810, "MotorControlDevRef"=w1805) -> ("MotorControlDevRef"=w1804:T5)  [unwired: 7 in, 1 out]
          n424 = call <vilib>:"Spark MAX Set Output Advanced.vi"("Control Mode"=Spark_MAX_Control_Type."Velocity", "Setpoint"=w1808, "MotorControlDevRef"=w1807) -> ("MotorControlDevRef"=w1806:T5)  [unwired: 7 in, 1 out]
        }
        frame #15 {
          n425 = Wait (ms)(milliseconds to wait=u32 1000) -> ()  [unwired: 1 out]
        }
        frame #16 {
          # "Shoot?"
          n426 = call "Feed to Shooter.vi"("Feed Input"=0.3) -> ()  [unwired: 11 in]
          n427 = Wait (ms)(milliseconds to wait=u32 2000) -> ()  [unwired: 1 out]
        }
        frame #17 {
          w1829 = 0.0 ("Output")
          # "Turn Off"
          n428 = call <vilib>:"WPI_MotorControlSetOutput.vi"("Output"=w1829, "MotorControlDevRef"=w1831) -> ()  [unwired: 7 in, 3 out]
          n429 = call <vilib>:"WPI_MotorControlSetOutput.vi"("Output"=w1829, "MotorControlDevRef"=w1830) -> ()  [unwired: 7 in, 3 out]
          n430 = call <vilib>:"WPI_RobotDriveArcadeDrive_Standard(NoSaturation).vi"("error in (no error)"=w1834, "Y axis value"=0.0, "X axis value"=0.0, "RobotDriveDevRef"=w1835) -> ()  [unwired: 8 out]
          n431 = Wait (ms)(milliseconds to wait=u32 1000) -> ()  [unwired: 1 out]
        }
        frame #18 {
          n432 = call <vilib>:"WPI_MotorControlSetOutput.vi"("Output"=0.0, "MotorControlDevRef"=w1839) -> ()  [unwired: 7 in, 3 out]
          n433 = call <vilib>:"WPI_MotorControlSetOutput.vi"("Output"=0.0, "MotorControlDevRef"=w1841) -> ()  [unwired: 7 in, 3 out]
        }
      }
    }
    frame "Turn Test" {
      n434 = flat-sequence {
        frame #0 {
          n435 = call <vilib>:"WPI_GyroRefNum Registry Get.vi"("refnum name"="AD Gyro") -> ("error out"=w1843:errorcluster, "GyroDevRef"=w1844:T14)  [unwired: 9 in]
          n436 = Wait (ms)(milliseconds to wait=u32 2000) -> ()  [unwired: 1 out]
          n437 = call <vilib>:"WPI_GyroReset.vi"("error in (no error)"=w1843, "GyroDevRef"=w1844) -> ()  [unwired: 8 in, 2 out]
        }
        frame #1 {
          n438 = while {
            stop <- w1848 stop-if-true
            n439 = call "Turn to Angle.vi"("Target Angle"=90.0) -> ("Angle Reached?"=w1848:bool)  [unwired: 10 in]
            n440 = Wait (ms)(milliseconds to wait=u32 10) -> ()  [unwired: 1 out]
          }
        }
      }
    }
    frame "Fender Shoot Move Shoot" {
      n441 = flat-sequence {
        tunnel: w1866 -> [w1875]
        tunnel: w1870 -> [w1876]
        tunnel: [w1876] -> w1851
        tunnel: [w1875] -> w1850
        tunnel: [w1878] -> w1871
        tunnel: [w1877] -> w1867
        tunnel: w1851 -> [w1878]
        tunnel: w1850 -> [w1877]
        tunnel: w1871 -> [w1883]
        tunnel: [w1883] -> w1869
        tunnel: [w1882] -> w1868
        tunnel: w1867 -> [w1882]
        tunnel: w1869 -> [w1895]
        tunnel: w1868 -> [w1894]
        tunnel: [w1889] -> w1855
        tunnel: [w1888] -> w1853
        tunnel: w1855 -> [w1898]
        tunnel: [w1898] -> w1854
        tunnel: w1853 -> [w1897]
        tunnel: [w1897] -> w1852
        tunnel: [w1901] -> w1859
        tunnel: w1854 -> [w1901]
        tunnel: [w1900] -> w1857
        tunnel: w1852 -> [w1900]
        tunnel: w1859 -> [w1904]
        tunnel: [w1904] -> w1858
        tunnel: w1857 -> [w1903]
        tunnel: [w1903] -> w1856
        tunnel: w1858 -> [w1917]
        tunnel: [w1916] -> w1863
        tunnel: w1856 -> [w1914]
        tunnel: [w1913] -> w1862
        tunnel: [w1924] -> w1873
        tunnel: [w1923] -> w1872
        tunnel: w1863 -> [w1921]
        tunnel: w1862 -> [w1920]
        tunnel: [w1921] -> w1865
        tunnel: [w1920] -> w1864
        tunnel: w1873 -> [w1935]
        tunnel: w1872 -> [w1934]
        tunnel: w1865 -> [w1931]
        tunnel: w1864 -> [w1932]
        tunnel: [w1932] -> w1861
        tunnel: [w1931] -> w1860
        tunnel: w1861 -> [w1941]
        tunnel: w1860 -> [w1939]
        frame #0 {
          n442 = Wait (ms)(milliseconds to wait=u32 500) -> ()  [unwired: 1 out]
        }
        frame #1 {
          n443 = while {
            stop <- TRUE stop-if-true
            n444 = call "Set Shooter Config.vi"("POV Joystick Input"=270) -> ()  [unwired: 3 in]
          }
          n445 = Wait (ms)(milliseconds to wait=u32 500) -> ()  [unwired: 1 out]
        }
        frame #2 {
          n446 = call <vilib>:"WPI_SolenoidRefNum Registry Get.vi"("refnum name"="Intake Pivot") -> ("error out"=w1887:errorcluster, "SolenoidDevRef"=w1886:T12)  [unwired: 9 in]
          n447 = call-poly <vilib>:"WPI_SolenoidSet.vi"("error in (no error)"=w1887, "Value"=WPI_SolenoidValue."Reverse", "SolenoidDevRef"=w1886) -> ()  [unwired: 7 in, 2 out]
        }
        frame #3 {
          n448 = global read "Global Shooter Speed.vi" "Shooter Speed Target"() -> (w1892:dbl)
          n449 = global read "Global Shooter Speed.vi" "Accelerator Speed Target"() -> (w1890:dbl)
          n450 = call <vilib>:"Spark MAX Set Output Advanced.vi"("Control Mode"=Spark_MAX_Control_Type."Velocity", "Setpoint"=w1892, "MotorControlDevRef"=w1895) -> ("MotorControlDevRef"=w1889:T5)  [unwired: 7 in, 1 out]
          n451 = call <vilib>:"Spark MAX Set Output Advanced.vi"("Control Mode"=Spark_MAX_Control_Type."Velocity", "Setpoint"=w1890, "MotorControlDevRef"=w1894) -> ("MotorControlDevRef"=w1888:T5)  [unwired: 7 in, 1 out]
        }
        frame #4 {
          n452 = Wait (ms)(milliseconds to wait=u32 3000) -> ()  [unwired: 1 out]
        }
        frame #5 {
          n453 = call "Feed to Shooter.vi"("Feed Input"=0.7) -> ()  [unwired: 11 in]
          n454 = Wait (ms)(milliseconds to wait=u32 2000) -> ()  [unwired: 1 out]
        }
        frame #6 {
          n455 = while {
            stop <- TRUE stop-if-true
            n456 = call "Set Shooter Config.vi"("POV Joystick Input"=0) -> ()  [unwired: 3 in]
          }
        }
        frame #7 {
          n457 = global read "Global Shooter Speed.vi" "Shooter Speed Target"() -> (w1912:dbl)
          n458 = global read "Global Shooter Speed.vi" "Accelerator Speed Target"() -> (w1908:dbl)
          n459 = Wait (ms)(milliseconds to wait=u32 1000) -> ()  [unwired: 1 out]
          n460 = Subtract(x=w1908, y=100.0) -> (x-y=w1909:dbl)
          n461 = Subtract(x=w1912, y=100.0) -> (x-y=w1910:dbl)
          n462 = call <vilib>:"Spark MAX Set Output Advanced.vi"("Control Mode"=Spark_MAX_Control_Type."Velocity", "Setpoint"=w1910, "MotorControlDevRef"=w1917) -> ("MotorControlDevRef"=w1916:T5)  [unwired: 7 in, 1 out]
          n463 = call <vilib>:"Spark MAX Set Output Advanced.vi"("Control Mode"=Spark_MAX_Control_Type."Velocity", "Setpoint"=w1909, "MotorControlDevRef"=w1914) -> ("MotorControlDevRef"=w1913:T5)  [unwired: 7 in, 1 out]
        }
        frame #8 {
          n464 = Wait (ms)(milliseconds to wait=u32 3000) -> ()  [unwired: 1 out]
          n465 = call <vilib>:"WPI_RobotDriveRefNum Registry Get.vi"("refnum name"="6MRobotDrive") -> ("error out"=w1927:errorcluster, "RobotDriveDevRef"=w1926:T4)  [unwired: 1 in, 8 out]
          n466 = call <vilib>:"WPI_RobotDriveArcadeDrive_Standard(NoSaturation).vi"("Y axis value"=0.0, "X axis value"=-0.5, "RobotDriveDevRef"=w1926) -> ()  [unwired: 1 in, 8 out]
          n467 = call <vilib>:"WPI_RobotDriveSafetyConfig.vi"("error in (no error)"=w1927, "mode"=WPI_SafetyOutputConfigMenu."Disable", "RobotDriveDevRef"=w1926) -> ("error out"=w1923:errorcluster, "RobotDriveDevRef"=w1924:T4)  [unwired: 7 in]
        }
        frame #9 {
          n468 = call <vilib>:"WPI_RobotDriveArcadeDrive_Standard(NoSaturation).vi"("error in (no error)"=w1934, "Y axis value"=0.0, "X axis value"=0.0, "RobotDriveDevRef"=w1935) -> ()  [unwired: 8 out]
          n469 = call "Feed to Shooter.vi"("Feed Input"=0.0) -> ()  [unwired: 11 in]
          n470 = Wait (ms)(milliseconds to wait=u32 1000) -> ()  [unwired: 1 out]
        }
        frame #10 {
          n471 = call <vilib>:"WPI_MotorControlSetOutput.vi"("Output"=0.0, "MotorControlDevRef"=w1939) -> ()  [unwired: 7 in, 3 out]
          n472 = call <vilib>:"WPI_MotorControlSetOutput.vi"("Output"=0.0, "MotorControlDevRef"=w1941) -> ()  [unwired: 7 in, 3 out]
        }
      }
    }
  }
